vi "(SubVI)DW7802.vi"() -> ()   [LabVIEW 2020]
uses:
  DW7912/Controls/(Ctrl)DW7912_Wave Seq.ctl
  System Command/Controls/(Ctrl)System Command_Trig GPIO Control.ctl
  Register Access/Controls/(Ctrl)Register Access_Cluster.ctl
  <vilib>/Utility/miscctls.llb/LVPointTypeDef.ctl
  Control Data/Controls/(Ctrl)Control Data_Save or Load Control Data_Function.ctl
  Libraries/GUI Log Class/GUI Log Class/Controls/line limit fgv enum.ctl
  Libraries/Haptic IC Class/Haptic IC/Haptic IC.lvclass/Haptic IC.ctl
  I2C/Controls/(Ctrl)I2C_8Bit_Read Array.ctl
  Waveform Editor/Controls/(Ctrl)Waveform Editor_Update Sampling Rate Value.ctl
  b2b9b553-3e13-44b6-91d2-097a3bc441c9.vi
  ce66826c-65e6-4b6c-9d2d-5a99ab5dd81e.vi
  a7fdcbe2-e318-4fc3-ac41-e38a3fe8abb3.vi
  Libraries/Haptic IC Class/Haptic IC/Accessors/Write freq ref.vi
  Libraries/Haptic IC Class/Haptic IC/Accessors/Write voltage range ref.vi
  Libraries/Haptic IC Class/Haptic IC/Accessors/Write mode ref.vi
  Variables/(Var)System Variables.vi
  I2C/Instance VIs/(SubVI)I2C_8Bit-8Bit_Read_Single.vi
  I2C/Instance VIs/(SubVI)I2C_8Bit-8Bit_Read_Sequential.vi
  I2C/Instance VIs/(SubVI)I2C_8Bit-8Bit_Read_Array.vi
  I2C/Instance VIs/(SubVI)I2C_8Bit-8Bit_Write_Single.vi
  I2C/Instance VIs/(SubVI)I2C_8Bit-8Bit_Write_Sequential.vi
  <vilib>/Comparison/Equal/Equal Functor/Equal Functor.lvclass
  Libraries/GUI Log Class/GUI Log Class/GUI Log Class.lvclass
  Libraries/Haptic IC Class/Haptic IC/Haptic IC.lvclass
panel:
  in  "MEM/AT_AB":T1={"OD Cycle"=2, "OD Level"=0, "OD Enable"=TRUE, "Shape"=0, "Enable"=FALSE, "Gain"=0} caption="BRAKE CTRL" {"Gain" items=["Auto", "X1.0", "X0.9", "X0.8", "X0.7", "X0.6", "X0.5", "X0.4"]; "OD Cycle" items=["4 Cycles", "6 Cycles", "8 Cycles", "10 Cycles"]; "OD Level" items=["X1.2", "X1.3", "X1.4", "X1.5"]; "Shape" items=["Square Wave", "Sine Wave"]}
  in  "Stop":bool
  in  "Read All":bool
  in  "Mode Tab":T2(tab)
  in  "Mem Set_Wave Seq Loop":T3 {"Loop 7" items=["X1", "X2", "X3", "X4", "X5", "X6", "X7", "X8", "X9", "X10", "X11", "X12", "X13", "X14", "X15", "Infinite"]; "Loop 6" items=["X1", "X2", "X3", "X4", "X5", "X6", "X7", "X8", "X9", "X10", "X11", "X12", "X13", "X14", "X15", "Infinite"]; "Loop 5" items=["X1", "X2", "X3", "X4", "X5", "X6", "X7", "X8", "X9", "X10", "X11", "X12", "X13", "X14", "X15", "Infinite"]; "Loop 4" items=["X1", "X2", "X3", "X4", "X5", "X6", "X7", "X8", "X9", "X10", "X11", "X12", "X13", "X14", "X15", "Infinite"]; "Loop 3" items=["X1", "X2", "X3", "X4", "X5", "X6", "X7", "X8", "X9", "X10", "X11", "X12", "X13", "X14", "X15", "Infinite"]; "Loop 2" items=["X1", "X2", "X3", "X4", "X5", "X6", "X7", "X8", "X9", "X10", "X11", "X12", "X13", "X14", "X15", "Infinite"]; "Loop 1" items=["X1", "X2", "X3", "X4", "X5", "X6", "X7", "X8", "X9", "X10", "X11", "X12", "X13", "X14", "X15", "Infinite"]; "Loop 0" items=["X1", "X2", "X3", "X4", "X5", "X6", "X7", "X8", "X9", "X10", "X11", "X12", "X13", "X14", "X15", "Infinite"]}
  in  "Mem_Stop":bool
  in  "Mem_Start":bool
  in  "Mem_Wave Seq":T5 caption="WAVE SEQUENCE" {"Wave Seq. 7"."Seq/Delay" items=["Empty", "1", "2", "3", "4", "5", "6", "7", "8", "9", "10", "11", "12", "13", "14", "15", "16", "17", "18", "19", "20", "21", "22", "23", "24", "25", "26", "27", "28", "29", "30", "31", "32", "33", "34", "35", "36", "37", "38", "39", "40", "41", "42", "43", "44", "45", "46", "47", "48", "49", "50", "51", "52", "53", "54", "55", "56", "57", "58", "59", "60", "61", "62", "63", "64", "65", "66", "67", "68", "69", "70", "71", "72", "73", "74", "75", "76", "77", "78", "79", "80", "81", "82", "83", "84", "85", "86", "87", "88", "89", "90", "91", "92", "93", "94", "95", "96", "97", "98", "99", "100", "101", "102", "103", "104", "105", "106", "107", "108", "109", "110", "111", "112", "113", "114", "115", "116", "117", "118", "119", "120", "121", "122", "123", "124", "125", "126", "127"]; "Wave Seq. 7"."Mode" items=["Wave Seq. 7", "Delay"]; "Wave Seq. 6"."Seq/Delay" items=["Empty", "1", "2", "3", "4", "5", "6", "7", "8", "9", "10", "11", "12", "13", "14", "15", "16", "17", "18", "19", "20", "21", "22", "23", "24", "25", "26", "27", "28", "29", "30", "31", "32", "33", "34", "35", "36", "37", "38", "39", "40", "41", "42", "43", "44", "45", "46", "47", "48", "49", "50", "51", "52", "53", "54", "55", "56", "57", "58", "59", "60", "61", "62", "63", "64", "65", "66", "67", "68", "69", "70", "71", "72", "73", "74", "75", "76", "77", "78", "79", "80", "81", "82", "83", "84", "85", "86", "87", "88", "89", "90", "91", "92", "93", "94", "95", "96", "97", "98", "99", "100", "101", "102", "103", "104", "105", "106", "107", "108", "109", "110", "111", "112", "113", "114", "115", "116", "117", "118", "119", "120", "121", "122", "123", "124", "125", "126", "127"]; "Wave Seq. 6"."Mode" items=["Wave Seq. 6", "Delay"]; "Wave Seq. 5"."Seq/Delay" items=["Empty", "1", "2", "3", "4", "5", "6", "7", "8", "9", "10", "11", "12", "13", "14", "15", "16", "17", "18", "19", "20", "21", "22", "23", "24", "25", "26", "27", "28", "29", "30", "31", "32", "33", "34", "35", "36", "37", "38", "39", "40", "41", "42", "43", "44", "45", "46", "47", "48", "49", "50", "51", "52", "53", "54", "55", "56", "57", "58", "59", "60", "61", "62", "63", "64", "65", "66", "67", "68", "69", "70", "71", "72", "73", "74", "75", "76", "77", "78", "79", "80", "81", "82", "83", "84", "85", "86", "87", "88", "89", "90", "91", "92", "93", "94", "95", "96", "97", "98", "99", "100", "101", "102", "103", "104", "105", "106", "107", "108", "109", "110", "111", "112", "113", "114", "115", "116", "117", "118", "119", "120", "121", "122", "123", "124", "125", "126", "127"]; "Wave Seq. 5"."Mode" items=["Wave Seq. 5", "Delay"]; "Wave Seq. 4"."Seq/Delay" items=["Empty", "1", "2", "3", "4", "5", "6", "7", "8", "9", "10", "11", "12", "13", "14", "15", "16", "17", "18", "19", "20", "21", "22", "23", "24", "25", "26", "27", "28", "29", "30", "31", "32", "33", "34", "35", "36", "37", "38", "39", "40", "41", "42", "43", "44", "45", "46", "47", "48", "49", "50", "51", "52", "53", "54", "55", "56", "57", "58", "59", "60", "61", "62", "63", "64", "65", "66", "67", "68", "69", "70", "71", "72", "73", "74", "75", "76", "77", "78", "79", "80", "81", "82", "83", "84", "85", "86", "87", "88", "89", "90", "91", "92", "93", "94", "95", "96", "97", "98", "99", "100", "101", "102", "103", "104", "105", "106", "107", "108", "109", "110", "111", "112", "113", "114", "115", "116", "117", "118", "119", "120", "121", "122", "123", "124", "125", "126", "127"]; "Wave Seq. 4"."Mode" items=["Wave Seq. 4", "Delay"]; "Wave Seq. 3"."Seq/Delay" items=["Empty", "1", "2", "3", "4", "5", "6", "7", "8", "9", "10", "11", "12", "13", "14", "15", "16", "17", "18", "19", "20", "21", "22", "23", "24", "25", "26", "27", "28", "29", "30", "31", "32", "33", "34", "35", "36", "37", "38", "39", "40", "41", "42", "43", "44", "45", "46", "47", "48", "49", "50", "51", "52", "53", "54", "55", "56", "57", "58", "59", "60", "61", "62", "63", "64", "65", "66", "67", "68", "69", "70", "71", "72", "73", "74", "75", "76", "77", "78", "79", "80", "81", "82", "83", "84", "85", "86", "87", "88", "89", "90", "91", "92", "93", "94", "95", "96", "97", "98", "99", "100", "101", "102", "103", "104", "105", "106", "107", "108", "109", "110", "111", "112", "113", "114", "115", "116", "117", "118", "119", "120", "121", "122", "123", "124", "125", "126", "127"]; "Wave Seq. 3"."Mode" items=["Wave Seq. 3", "Delay"]; "Wave Seq. 2"."Seq/Delay" items=["Empty", "1", "2", "3", "4", "5", "6", "7", "8", "9", "10", "11", "12", "13", "14", "15", "16", "17", "18", "19", "20", "21", "22", "23", "24", "25", "26", "27", "28", "29", "30", "31", "32", "33", "34", "35", "36", "37", "38", "39", "40", "41", "42", "43", "44", "45", "46", "47", "48", "49", "50", "51", "52", "53", "54", "55", "56", "57", "58", "59", "60", "61", "62", "63", "64", "65", "66", "67", "68", "69", "70", "71", "72", "73", "74", "75", "76", "77", "78", "79", "80", "81", "82", "83", "84", "85", "86", "87", "88", "89", "90", "91", "92", "93", "94", "95", "96", "97", "98", "99", "100", "101", "102", "103", "104", "105", "106", "107", "108", "109", "110", "111", "112", "113", "114", "115", "116", "117", "118", "119", "120", "121", "122", "123", "124", "125", "126", "127"]; "Wave Seq. 2"."Mode" items=["Wave Seq. 2", "Delay"]; "Wave Seq. 1"."Seq/Delay" items=["Empty", "1", "2", "3", "4", "5", "6", "7", "8", "9", "10", "11", "12", "13", "14", "15", "16", "17", "18", "19", "20", "21", "22", "23", "24", "25", "26", "27", "28", "29", "30", "31", "32", "33", "34", "35", "36", "37", "38", "39", "40", "41", "42", "43", "44", "45", "46", "47", "48", "49", "50", "51", "52", "53", "54", "55", "56", "57", "58", "59", "60", "61", "62", "63", "64", "65", "66", "67", "68", "69", "70", "71", "72", "73", "74", "75", "76", "77", "78", "79", "80", "81", "82", "83", "84", "85", "86", "87", "88", "89", "90", "91", "92", "93", "94", "95", "96", "97", "98", "99", "100", "101", "102", "103", "104", "105", "106", "107", "108", "109", "110", "111", "112", "113", "114", "115", "116", "117", "118", "119", "120", "121", "122", "123", "124", "125", "126", "127"]; "Wave Seq. 1"."Mode" items=["Wave Seq. 1", "Delay"]; "Wave Seq. 0"."Seq/Delay" items=["Empty", "1", "2", "3", "4", "5", "6", "7", "8", "9", "10", "11", "12", "13", "14", "15", "16", "17", "18", "19", "20", "21", "22", "23", "24", "25", "26", "27", "28", "29", "30", "31", "32", "33", "34", "35", "36", "37", "38", "39", "40", "41", "42", "43", "44", "45", "46", "47", "48", "49", "50", "51", "52", "53", "54", "55", "56", "57", "58", "59", "60", "61", "62", "63", "64", "65", "66", "67", "68", "69", "70", "71", "72", "73", "74", "75", "76", "77", "78", "79", "80", "81", "82", "83", "84", "85", "86", "87", "88", "89", "90", "91", "92", "93", "94", "95", "96", "97", "98", "99", "100", "101", "102", "103", "104", "105", "106", "107", "108", "109", "110", "111", "112", "113", "114", "115", "116", "117", "118", "119", "120", "121", "122", "123", "124", "125", "126", "127"]; "Wave Seq. 0"."Mode" items=["Wave Seq. 0", "Delay"]}
  in  "Mem_Main Seq Loop":u8(ring) caption="Sequence Loop" items=["X1", "X2", "X3", "X4", "X5", "X6", "X7", "X8", "X9", "X10", "X11", "X12", "X13", "X14", "X15", "Infinite"]
  in  "Mem_Read":bool caption="Memory Mode"
  in  "Com_Bst_Mem Gain":u8(ring) caption="MEM Gain" items=["100%", "87.5%", "75%", "62.5%", "50%", "37.5%", "25%", "12.5%"]
  in  "Com_Bst_Mute":bool
  in  "AT_Track_OD Cycle":u8(ring)=2 caption="Over Drive Cycle" items=["4 Cycles", "6 Cycles", "8 Cycles", "10 Cycles"]
  in  "AT_Track_OD Level":u8(ring) caption="Over Drive Level" items=["X1.2", "X1.3", "X1.4", "X1.5"]
  in  "AT_Track_OD Enable":bool=TRUE
  in  "AT_Track_Shape":u8(ring) caption="Track Shape" items=["Square Wave", "Sine Wave"]
  in  "AT_Track_Idle":u8(ring)=3 caption="Track Idle" items=["10.66ms", "21.32ms", "31.98ms", "42.64ms", "53.30ms", "63.96ms", "74.62ms", "85.28ms", "95.94ms", "106.60ms", "117.26ms", "127.92ms", "138.58ms", "149.24ms", "159.90ms", "170.56ms", "181.22ms", "191.88ms", "202.54ms", "213.20ms", "223.86ms", "234.52ms", "245.18ms", "255.84ms", "266.50ms", "277.16ms", "287.82ms", "298.48ms", "309.14ms", "319.80ms", "330.46ms", "341.12ms", "351.78ms", "362.44ms", "373.10ms", "383.76ms", "394.42ms", "405.08ms", "415.74ms", "426.40ms", "437.06ms", "447.72ms", "458.38ms", "469.04ms", "479.70ms", "490.36ms", "501.02ms", "511.68ms", "522.34ms", "533.00ms", "543.66ms", "554.32ms", "564.98ms", "575.64ms", "586.30ms", "596.96ms", "607.62ms", "618.28ms", "628.94ms", "639.60ms", "650.26ms", "660.92ms", "671.58ms", "682.24ms", "692.90ms", "703.56ms", "714.22ms", "724.88ms", "735.54ms", "746.20ms", "756.86ms", "767.52ms", "778.18ms", "788.84ms", "799.50ms", "810.16ms", "820.82ms", "831.48ms", "842.14ms", "852.80ms", "863.46ms", "874.12ms", "884.78ms", "895.44ms", "906.10ms", "916.76ms", "927.42ms", "938.08ms", "948.74ms", "959.40ms", "970.06ms", "980.72ms", "991.38ms", "1002.04ms", "1012.70ms", "1023.36ms", "1034.02ms", "1044.68ms", "1055.34ms", "1066.00ms", "1076.66ms", "1087.32ms", "1097.98ms", "1108.64ms", "1119.30ms", "1129.96ms", "1140.62ms", "1151.28ms", "1161.94ms", "1172.60ms", "1183.26ms", "1193.92ms", "1204.58ms", "1215.24ms", "1225.90ms", "1236.56ms", "1247.22ms", "1257.88ms", "1268.54ms", "1279.20ms", "1289.86ms", "1300.52ms", "1311.18ms", "1321.84ms", "1332.50ms", "1343.16ms", "1353.82ms", "1364.48ms", "1375.14ms", "1385.80ms", "1396.46ms", "1407.12ms", "1417.78ms", "1428.44ms", "1439.10ms", "1449.76ms", "1460.42ms", "1471.08ms", "1481.74ms", "1492.40ms", "1503.06ms", "1513.72ms", "1524.38ms", "1535.04ms", "1545.70ms", "1556.36ms", "1567.02ms", "1577.68ms", "1588.34ms", "1599.00ms", "1609.66ms", "1620.32ms", "1630.98ms", "1641.64ms", "1652.30ms", "1662.96ms", "1673.62ms", "1684.28ms", "1694.94ms", "1705.60ms", "1716.26ms", "1726.92ms", "1737.58ms", "1748.24ms", "1758.90ms", "1769.56ms", "1780.22ms", "1790.88ms", "1801.54ms", "1812.20ms", "1822.86ms", "1833.52ms", "1844.18ms", "1854.84ms", "1865.50ms", "1876.16ms", "1886.82ms", "1897.48ms", "1908.14ms", "1918.80ms", "1929.46ms", "1940.12ms", "1950.78ms", "1961.44ms", "1972.10ms", "1982.76ms", "1993.42ms", "2004.08ms", "2014.74ms", "2025.40ms", "2036.06ms", "2046.72ms", "2057.38ms", "2068.04ms", "2078.70ms", "2089.36ms", "2100.02ms", "2110.68ms", "2121.34ms", "2132.00ms", "2142.66ms", "2153.32ms", "2163.98ms", "2174.64ms", "2185.30ms", "2195.96ms", "2206.62ms", "2217.28ms", "2227.94ms", "2238.60ms", "2249.26ms", "2259.92ms", "2270.58ms", "2281.24ms", "2291.90ms", "2302.56ms", "2313.22ms", "2323.88ms", "2334.54ms", "2345.20ms", "2355.86ms", "2366.52ms", "2377.18ms", "2387.84ms", "2398.50ms", "2409.16ms", "2419.82ms", "2430.48ms", "2441.14ms", "2451.80ms", "2462.46ms", "2473.12ms", "2483.78ms", "2494.44ms", "2505.10ms", "2515.76ms", "2526.42ms", "2537.08ms", "2547.74ms", "2558.40ms", "2569.06ms", "2579.72ms", "2590.38ms", "2601.04ms", "2611.70ms", "2622.36ms", "2633.02ms", "2643.68ms", "2654.34ms", "2665.00ms", "2675.66ms", "2686.32ms", "2696.98ms", "2707.64ms", "2718.30ms", "2728.96ms"]
  in  "AT_Track_Play":u8(ring)=128 caption="Track Play" items=["10.66ms", "21.32ms", "31.98ms", "42.64ms", "53.30ms", "63.96ms", "74.62ms", "85.28ms", "95.94ms", "106.60ms", "117.26ms", "127.92ms", "138.58ms", "149.24ms", "159.90ms", "170.56ms", "181.22ms", "191.88ms", "202.54ms", "213.20ms", "223.86ms", "234.52ms", "245.18ms", "255.84ms", "266.50ms", "277.16ms", "287.82ms", "298.48ms", "309.14ms", "319.80ms", "330.46ms", "341.12ms", "351.78ms", "362.44ms", "373.10ms", "383.76ms", "394.42ms", "405.08ms", "415.74ms", "426.40ms", "437.06ms", "447.72ms", "458.38ms", "469.04ms", "479.70ms", "490.36ms", "501.02ms", "511.68ms", "522.34ms", "533.00ms", "543.66ms", "554.32ms", "564.98ms", "575.64ms", "586.30ms", "596.96ms", "607.62ms", "618.28ms", "628.94ms", "639.60ms", "650.26ms", "660.92ms", "671.58ms", "682.24ms", "692.90ms", "703.56ms", "714.22ms", "724.88ms", "735.54ms", "746.20ms", "756.86ms", "767.52ms", "778.18ms", "788.84ms", "799.50ms", "810.16ms", "820.82ms", "831.48ms", "842.14ms", "852.80ms", "863.46ms", "874.12ms", "884.78ms", "895.44ms", "906.10ms", "916.76ms", "927.42ms", "938.08ms", "948.74ms", "959.40ms", "970.06ms", "980.72ms", "991.38ms", "1002.04ms", "1012.70ms", "1023.36ms", "1034.02ms", "1044.68ms", "1055.34ms", "1066.00ms", "1076.66ms", "1087.32ms", "1097.98ms", "1108.64ms", "1119.30ms", "1129.96ms", "1140.62ms", "1151.28ms", "1161.94ms", "1172.60ms", "1183.26ms", "1193.92ms", "1204.58ms", "1215.24ms", "1225.90ms", "1236.56ms", "1247.22ms", "1257.88ms", "1268.54ms", "1279.20ms", "1289.86ms", "1300.52ms", "1311.18ms", "1321.84ms", "1332.50ms", "1343.16ms", "1353.82ms", "1364.48ms", "1375.14ms", "1385.80ms", "1396.46ms", "1407.12ms", "1417.78ms", "1428.44ms", "1439.10ms", "1449.76ms", "1460.42ms", "1471.08ms", "1481.74ms", "1492.40ms", "1503.06ms", "1513.72ms", "1524.38ms", "1535.04ms", "1545.70ms", "1556.36ms", "1567.02ms", "1577.68ms", "1588.34ms", "1599.00ms", "1609.66ms", "1620.32ms", "1630.98ms", "1641.64ms", "1652.30ms", "1662.96ms", "1673.62ms", "1684.28ms", "1694.94ms", "1705.60ms", "1716.26ms", "1726.92ms", "1737.58ms", "1748.24ms", "1758.90ms", "1769.56ms", "1780.22ms", "1790.88ms", "1801.54ms", "1812.20ms", "1822.86ms", "1833.52ms", "1844.18ms", "1854.84ms", "1865.50ms", "1876.16ms", "1886.82ms", "1897.48ms", "1908.14ms", "1918.80ms", "1929.46ms", "1940.12ms", "1950.78ms", "1961.44ms", "1972.10ms", "1982.76ms", "1993.42ms", "2004.08ms", "2014.74ms", "2025.40ms", "2036.06ms", "2046.72ms", "2057.38ms", "2068.04ms", "2078.70ms", "2089.36ms", "2100.02ms", "2110.68ms", "2121.34ms", "2132.00ms", "2142.66ms", "2153.32ms", "2163.98ms", "2174.64ms", "2185.30ms", "2195.96ms", "2206.62ms", "2217.28ms", "2227.94ms", "2238.60ms", "2249.26ms", "2259.92ms", "2270.58ms", "2281.24ms", "2291.90ms", "2302.56ms", "2313.22ms", "2323.88ms", "2334.54ms", "2345.20ms", "2355.86ms", "2366.52ms", "2377.18ms", "2387.84ms", "2398.50ms", "2409.16ms", "2419.82ms", "2430.48ms", "2441.14ms", "2451.80ms", "2462.46ms", "2473.12ms", "2483.78ms", "2494.44ms", "2505.10ms", "2515.76ms", "2526.42ms", "2537.08ms", "2547.74ms", "2558.40ms", "2569.06ms", "2579.72ms", "2590.38ms", "2601.04ms", "2611.70ms", "2622.36ms", "2633.02ms", "2643.68ms", "2654.34ms", "2665.00ms", "2675.66ms", "2686.32ms", "2696.98ms", "2707.64ms", "2718.30ms", "Infinite"]
  in  "AT_Track_Loop":u8(ring) caption="Track Loop" items=["X1", "X2", "X3", "X4", "X5", "X6", "X7", "X8", "X9", "X10", "X11", "X12", "X13", "X14", "X15", "Infinite"]
  in  "AT_Track_Pattern":bool=TRUE
  in  "AT_Read":bool caption="Auto Track Mode"
  in  "AT_Start":bool
  in  "AT_Stop":bool
  in  "Trig_Wave_F_Enable":bool=TRUE
  in  "Trig_Wave_R_Enable":bool=TRUE
  in  "Trig_Wave_F":u8(ring) caption="TRIG F Wave" items=["Empty", "1", "2", "3", "4", "5", "6", "7", "8", "9", "10", "11", "12", "13", "14", "15", "16", "17", "18", "19", "20", "21", "22", "23", "24", "25", "26", "27", "28", "29", "30", "31", "32", "33", "34", "35", "36", "37", "38", "39", "40", "41", "42", "43", "44", "45", "46", "47", "48", "49", "50", "51", "52", "53", "54", "55", "56", "57", "58", "59", "60", "61", "62", "63", "64", "65", "66", "67", "68", "69", "70", "71", "72", "73", "74", "75", "76", "77", "78", "79", "80", "81", "82", "83", "84", "85", "86", "87", "88", "89", "90", "91", "92", "93", "94", "95", "96", "97", "98", "99", "100", "101", "102", "103", "104", "105", "106", "107", "108", "109", "110", "111", "112", "113", "114", "115", "116", "117", "118", "119", "120", "121", "122", "123", "124", "125", "126", "127"]
  in  "Trig_Wave_R":u8(ring) caption="TRIG R Wave" items=["Empty", "1", "2", "3", "4", "5", "6", "7", "8", "9", "10", "11", "12", "13", "14", "15", "16", "17", "18", "19", "20", "21", "22", "23", "24", "25", "26", "27", "28", "29", "30", "31", "32", "33", "34", "35", "36", "37", "38", "39", "40", "41", "42", "43", "44", "45", "46", "47", "48", "49", "50", "51", "52", "53", "54", "55", "56", "57", "58", "59", "60", "61", "62", "63", "64", "65", "66", "67", "68", "69", "70", "71", "72", "73", "74", "75", "76", "77", "78", "79", "80", "81", "82", "83", "84", "85", "86", "87", "88", "89", "90", "91", "92", "93", "94", "95", "96", "97", "98", "99", "100", "101", "102", "103", "104", "105", "106", "107", "108", "109", "110", "111", "112", "113", "114", "115", "116", "117", "118", "119", "120", "121", "122", "123", "124", "125", "126", "127"]
  out "Trig_Gen_Pict":picture
  in  "Trig_Ctrl_Interval":u8(ring)=4 caption="TRIG Interval" items=["2.5ms", "5ms", "10ms", "20ms", "40ms", "60ms", "80ms", "100ms"]
  in  "Trig_Ctrl_Tirg Mode":bool=TRUE
  in  "Trig_Ctrl_Restart Enable":bool
  in  "Trig_Ctrl_Trig Level":bool
  in  "Trig_Ctrl_Trig Priority":bool
  in  "Trig_Gen_Set":bool
  in  "Trig_Gen_Setting":T6={"1st Trig"={"Trigger"=TRUE, "Low"=0, "High"=100}, "2nd Trig"={"Trigger"=FALSE, "Low"=0, "High"=100}, "3rd Trig"={"Trigger"=FALSE, "Low"=0, "High"=100}, "4th Trig"={"Trigger"=FALSE, "Low"=0, "High"=1}} {"4th Trig"."High" min=1 max=8000; "4th Trig"."Low" max=7999; "3rd Trig"."High" min=1 max=8000; "3rd Trig"."Low" max=7999; "2nd Trig"."High" min=1 max=8000; "2nd Trig"."Low" max=7999; "1st Trig"."High" min=1 max=8000; "1st Trig"."Low" max=7999}
  in  "Trig_Read":bool caption="Trig Mode"
  in  "Common Tab":T7(tab)
  in  "Com_ACT_CAL F0":bool
  in  "Com_ACT_F0 In":u16(ring)=180 caption="ACT F0 In" items=["0Hz", "1Hz", "2Hz", "3Hz", "4Hz", "5Hz", "6Hz", "7Hz", "8Hz", "9Hz", "10Hz", "11Hz", "12Hz", "13Hz", "14Hz", "15Hz", "16Hz", "17Hz", "18Hz", "19Hz", "20Hz", "21Hz", "22Hz", "23Hz", "24Hz", "25Hz", "26Hz", "27Hz", "28Hz", "29Hz", "30Hz", "31Hz", "32Hz", "33Hz", "34Hz", "35Hz", "36Hz", "37Hz", "38Hz", "39Hz", "40Hz", "41Hz", "42Hz", "43Hz", "44Hz", "45Hz", "46Hz", "47Hz", "48Hz", "49Hz", "50Hz", "51Hz", "52Hz", "53Hz", "54Hz", "55Hz", "56Hz", "57Hz", "58Hz", "59Hz", "60Hz", "61Hz", "62Hz", "63Hz", "64Hz", "65Hz", "66Hz", "67Hz", "68Hz", "69Hz", "70Hz", "71Hz", "72Hz", "73Hz", "74Hz", "75Hz", "76Hz", "77Hz", "78Hz", "79Hz", "80Hz", "81Hz", "82Hz", "83Hz", "84Hz", "85Hz", "86Hz", "87Hz", "88Hz", "89Hz", "90Hz", "91Hz", "92Hz", "93Hz", "94Hz", "95Hz", "96Hz", "97Hz", "98Hz", "99Hz", "100Hz", "101Hz", "102Hz", "103Hz", "104Hz", "105Hz", "106Hz", "107Hz", "108Hz", "109Hz", "110Hz", "111Hz", "112Hz", "113Hz", "114Hz", "115Hz", "116Hz", "117Hz", "118Hz", "119Hz", "120Hz", "121Hz", "122Hz", "123Hz", "124Hz", "125Hz", "126Hz", "127Hz", "128Hz", "129Hz", "130Hz", "131Hz", "132Hz", "133Hz", "134Hz", "135Hz", "136Hz", "137Hz", "138Hz", "139Hz", "140Hz", "141Hz", "142Hz", "143Hz", "144Hz", "145Hz", "146Hz", "147Hz", "148Hz", "149Hz", "150Hz", "151Hz", "152Hz", "153Hz", "154Hz", "155Hz", "156Hz", "157Hz", "158Hz", "159Hz", "160Hz", "161Hz", "162Hz", "163Hz", "164Hz", "165Hz", "166Hz", "167Hz", "168Hz", "169Hz", "170Hz", "171Hz", "172Hz", "173Hz", "174Hz", "175Hz", "176Hz", "177Hz", "178Hz", "179Hz", "180Hz", "181Hz", "182Hz", "183Hz", "184Hz", "185Hz", "186Hz", "187Hz", "188Hz", "189Hz", "190Hz", "191Hz", "192Hz", "193Hz", "194Hz", "195Hz", "196Hz", "197Hz", "198Hz", "199Hz", "200Hz", "201Hz", "202Hz", "203Hz", "204Hz", "205Hz", "206Hz", "207Hz", "208Hz", "209Hz", "210Hz", "211Hz", "212Hz", "213Hz", "214Hz", "215Hz", "216Hz", "217Hz", "218Hz", "219Hz", "220Hz", "221Hz", "222Hz", "223Hz", "224Hz", "225Hz", "226Hz", "227Hz", "228Hz", "229Hz", "230Hz", "231Hz", "232Hz", "233Hz", "234Hz", "235Hz", "236Hz", "237Hz", "238Hz", "239Hz", "240Hz", "241Hz", "242Hz", "243Hz", "244Hz", "245Hz", "246Hz", "247Hz", "248Hz", "249Hz", "250Hz", "251Hz", "252Hz", "253Hz", "254Hz", "255Hz", "256Hz", "257Hz", "258Hz", "259Hz", "260Hz", "261Hz", "262Hz", "263Hz", "264Hz", "265Hz", "266Hz", "267Hz", "268Hz", "269Hz", "270Hz", "271Hz", "272Hz", "273Hz", "274Hz", "275Hz", "276Hz", "277Hz", "278Hz", "279Hz", "280Hz", "281Hz", "282Hz", "283Hz", "284Hz", "285Hz", "286Hz", "287Hz", "288Hz", "289Hz", "290Hz", "291Hz", "292Hz", "293Hz", "294Hz", "295Hz", "296Hz", "297Hz", "298Hz", "299Hz", "300Hz", "301Hz", "302Hz", "303Hz", "304Hz", "305Hz", "306Hz", "307Hz", "308Hz", "309Hz", "310Hz", "311Hz", "312Hz", "313Hz", "314Hz", "315Hz", "316Hz", "317Hz", "318Hz", "319Hz", "320Hz", "321Hz", "322Hz", "323Hz", "324Hz", "325Hz", "326Hz", "327Hz", "328Hz", "329Hz", "330Hz", "331Hz", "332Hz", "333Hz", "334Hz", "335Hz", "336Hz", "337Hz", "338Hz", "339Hz", "340Hz", "341Hz", "342Hz", "343Hz", "344Hz", "345Hz", "346Hz", "347Hz", "348Hz", "349Hz", "350Hz", "351Hz", "352Hz", "353Hz", "354Hz", "355Hz", "356Hz", "357Hz", "358Hz", "359Hz", "360Hz", "361Hz", "362Hz", "363Hz", "364Hz", "365Hz", "366Hz", "367Hz", "368Hz", "369Hz", "370Hz", "371Hz", "372Hz", "373Hz", "374Hz", "375Hz", "376Hz", "377Hz", "378Hz", "379Hz", "380Hz", "381Hz", "382Hz", "383Hz", "384Hz", "385Hz", "386Hz", "387Hz", "388Hz", "389Hz", "390Hz", "391Hz", "392Hz", "393Hz", "394Hz", "395Hz", "396Hz", "397Hz", "398Hz", "399Hz", "400Hz", "401Hz", "402Hz", "403Hz", "404Hz", "405Hz", "406Hz", "407Hz", "408Hz", "409Hz", "410Hz", "411Hz", "412Hz", "413Hz", "414Hz", "415Hz", "416Hz", "417Hz", "418Hz", "419Hz", "420Hz", "421Hz", "422Hz", "423Hz", "424Hz", "425Hz", "426Hz", "427Hz", "428Hz", "429Hz", "430Hz", "431Hz", "432Hz", "433Hz", "434Hz", "435Hz", "436Hz", "437Hz", "438Hz", "439Hz", "440Hz", "441Hz", "442Hz", "443Hz", "444Hz", "445Hz", "446Hz", "447Hz", "448Hz", "449Hz", "450Hz", "451Hz", "452Hz", "453Hz", "454Hz", "455Hz", "456Hz", "457Hz", "458Hz", "459Hz", "460Hz", "461Hz", "462Hz", "463Hz", "464Hz", "465Hz", "466Hz", "467Hz", "468Hz", "469Hz", "470Hz", "471Hz", "472Hz", "473Hz", "474Hz", "475Hz", "476Hz", "477Hz", "478Hz", "479Hz", "480Hz", "481Hz", "482Hz", "483Hz", "484Hz", "485Hz", "486Hz", "487Hz", "488Hz", "489Hz", "490Hz", "491Hz", "492Hz", "493Hz", "494Hz", "495Hz", "496Hz", "497Hz", "498Hz", "499Hz", "500Hz", "501Hz", "502Hz", "503Hz", "504Hz", "505Hz", "506Hz", "507Hz", "508Hz", "509Hz", "510Hz", "511Hz"]
  in  "Com_ACT_Freq Range":u16(ring)=1 caption="Freq Range" items=["±20%", "±15%", "±10%", "±5%"]
  in  "Com_Mode_Trig Enable":bool
  in  "Com_Mode_Int Enable":bool
  in  "Com_Mode_Play Mode":u8(ring)=2 caption="Play Mode" items=["MEM Mode", "RTP Mode", "Auto Track Mode", "DIAG Mode"]
  out "Com_Status_Result":string caption="Result"
  in  "Com_VD Clamp":u8(ring)=85 caption="VD Clamp" items=["0.000V", "0.024V", "0.048V", "0.072V", "0.096V", "0.120V", "0.144V", "0.168V", "0.192V", "0.216V", "0.240V", "0.264V", "0.288V", "0.312V", "0.336V", "0.360V", "0.384V", "0.408V", "0.432V", "0.456V", "0.480V", "0.504V", "0.528V", "0.552V", "0.576V", "0.600V", "0.624V", "0.648V", "0.672V", "0.696V", "0.720V", "0.744V", "0.768V", "0.792V", "0.816V", "0.840V", "0.864V", "0.888V", "0.912V", "0.936V", "0.960V", "0.984V", "1.008V", "1.032V", "1.056V", "1.080V", "1.104V", "1.128V", "1.152V", "1.176V", "1.200V", "1.224V", "1.248V", "1.272V", "1.296V", "1.320V", "1.344V", "1.368V", "1.392V", "1.416V", "1.440V", "1.464V", "1.488V", "1.512V", "1.536V", "1.560V", "1.584V", "1.608V", "1.632V", "1.656V", "1.680V", "1.704V", "1.728V", "1.752V", "1.776V", "1.800V", "1.824V", "1.848V", "1.872V", "1.896V", "1.920V", "1.944V", "1.968V", "1.992V", "2.016V", "2.040V", "2.064V", "2.088V", "2.112V", "2.136V", "2.160V", "2.184V", "2.208V", "2.232V", "2.256V", "2.280V", "2.304V", "2.328V", "2.352V", "2.376V", "2.400V", "2.424V", "2.448V", "2.472V", "2.496V", "2.520V", "2.544V", "2.568V", "2.592V", "2.616V", "2.640V", "2.664V", "2.688V", "2.712V", "2.736V", "2.760V", "2.784V", "2.808V", "2.832V", "2.856V", "2.880V", "2.904V", "2.928V", "2.952V", "2.976V", "3.000V", "3.024V", "3.048V", "3.072V", "3.096V", "3.120V", "3.144V", "3.168V", "3.192V", "3.216V", "3.240V", "3.264V", "3.288V", "3.312V", "3.336V", "3.360V", "3.384V", "3.408V", "3.432V", "3.456V", "3.480V", "3.504V", "3.528V", "3.552V", "3.576V", "3.600V", "3.624V", "3.648V", "3.672V", "3.696V", "3.720V", "3.744V", "3.768V", "3.792V", "3.816V", "3.840V", "3.864V", "3.888V", "3.912V", "3.936V", "3.960V", "3.984V", "4.008V", "4.032V", "4.056V", "4.080V", "4.104V", "4.128V", "4.152V", "4.176V", "4.200V", "4.224V", "4.248V", "4.272V", "4.296V", "4.320V", "4.344V", "4.368V", "4.392V", "4.416V", "4.440V", "4.464V", "4.488V", "4.512V", "4.536V", "4.560V", "4.584V", "4.608V", "4.632V", "4.656V", "4.680V", "4.704V", "4.728V", "4.752V", "4.776V", "4.800V", "4.824V", "4.848V", "4.872V", "4.896V", "4.920V", "4.944V", "4.968V", "4.992V", "5.016V", "5.040V", "5.064V", "5.088V", "5.112V", "5.136V", "5.160V", "5.184V", "5.208V", "5.232V", "5.256V", "5.280V", "5.304V", "5.328V", "5.352V", "5.376V", "5.400V", "5.424V", "5.448V", "5.472V", "5.496V", "5.520V", "5.544V", "5.568V", "5.592V", "5.616V", "5.640V", "5.664V", "5.688V", "5.712V", "5.736V", "5.760V", "5.784V", "5.808V", "5.832V", "5.856V", "5.880V", "5.904V", "5.928V", "5.952V", "5.976V", "6.000V", "6.024V", "6.048V", "6.072V", "6.096V", "6.120V"]
  in  "Com_PWM_Mode":u8(ring) caption="VD Clamp Reg" items=["Header", "VD Clamp"]
  in  "Com_PWM_Freq":u8(ring)=2 caption="PWM Freq." items=["12kHz", "24kHz", "48kHz", "48kHz"]
  in  "Com_Status_Select":T8(ring) caption="Select"
  in  "Com_Read":bool caption="Common"
  in  "Com 2_Reset_SWRST":bool
  in  "Com 2_FIFO_Empty Level":u16=256 caption="Empty Level" max=6144
  in  "Com 2_FIFO_Full Level":u16=1792 caption="Full Level" max=6144
  in  "Com 2_FIFO_Size":u16=2048 caption="FIFO Size" max=6144
  in  "Com 2_ZXD_Sense Time":u8(ring)=2 caption="Sense Time" items=["50us", "100us", "150us", "200us"]
  in  "Com 2_ZXD_BEMF Gain":u8(ring)=10 caption="BEMF Gain" items=["1x", "2x", "3x", "4x", "5x", "6x", "8x", "10x", "20x", "30x", "40x", "50x", "60x", "80x", "100x", "120x"]
  in  "Com 2_ZXD_GND Time":u8(ring)=3 caption="GND Time" items=["25us", "50us", "75us", "100us", "125us", "150us", "175us", "200us", "225us", "250us", "275us", "300us", "325us", "350us", "375us", "400us"]
  in  "Com 2_ZXD_Null Time":u8(ring)=3 caption="Null Time" items=["25us", "50us", "75us", "100us", "125us", "150us", "175us", "200us", "225us", "250us", "275us", "300us", "325us", "350us", "375us", "400us"]
  in  "Com 2_INTZ":T9={"OCP"=TRUE, "TSD"=TRUE, "UVLO"=TRUE, "FIFO_EMPTY"=TRUE, "FIFO_FULL"=TRUE, "ACT_OPEN"=TRUE, "ACT_SHORT"=TRUE} caption="INTZ_MASK"
  in  "Com 2_Read":bool caption="Common 2"
  in  "Hidden_Register Access":T11={"Register 1"={"Addr"=64, "Name"="TRACK_CONFIG", "Data Size"=1, "R Data"=0, "R Btn"=FALSE, "W Data"=147, "W Btn"=FALSE}, "Register 2"={"Addr"=65, "Name"="BRAKE_CTRL", "Data Size"=1, "R Data"=0, "R Btn"=FALSE, "W Data"=2, "W Btn"=FALSE}, "Register 3"={"Addr"=66, "Name"="BEMF_VTH/VTL", "Data Size"=1, "R Data"=0, "R Btn"=FALSE, "W Data"=17, "W Btn"=FALSE}, "Register 4"={"Addr"=67, "Name"="BEMF_MAX", "Data Size"=1, "R Data"=0, "R Btn"=FALSE, "W Data"=0, "W Btn"=FALSE}, "Register 5"={"Addr"=68, "Name"="BEMF_MIN", "Data Size"=1, "R Data"=0, "R Btn"=FALSE, "W Data"=0, "W Btn"=FALSE}, "Register 6"={"Addr"=69, "Name"="VCOM", "Data Size"=1, "R Data"=0, "R Btn"=FALSE, "W Data"=0, "W Btn"=FALSE}, "Register 7"={"Addr"=70, "Name"="ACT_CNT", "Data Size"=2, "R Data"=0, "R Btn"=FALSE, "W Data"=0, "W Btn"=FALSE}, "Register 8"={"Addr"=72, "Name"="QTZ_CNT", "Data Size"=2, "R Data"=0, "R Btn"=FALSE, "W Data"=0, "W Btn"=FALSE}, "Register 9"={"Addr"=74, "Name"="ACT_RES_M", "Data Size"=2, "R Data"=0, "R Btn"=FALSE, "W Data"=0, "W Btn"=FALSE}, "Register 10"={"Addr"=76, "Name"="REF_RES", "Data Size"=2, "R Data"=0, "R Btn"=FALSE, "W Data"=0, "W Btn"=FALSE}, "Register 11"={"Addr"=78, "Name"="PROTECTION_ON", "Data Size"=1, "R Data"=0, "R Btn"=FALSE, "W Data"=2, "W Btn"=FALSE}, "Register 12"={"Addr"=79, "Name"="PROTECTION_OFF", "Data Size"=1, "R Data"=0, "R Btn"=FALSE, "W Data"=120, "W Btn"=FALSE}, "Register 13"={"Addr"=0, "Name"="", "Data Size"=1, "R Data"=0, "R Btn"=FALSE, "W Data"=0, "W Btn"=FALSE}, "Register 14"={"Addr"=96, "Name"="TRACK_CONFIG", "Data Size"=1, "R Data"=0, "R Btn"=FALSE, "W Data"=3, "W Btn"=FALSE}, "Register 15"={"Addr"=97, "Name"="BRAKE_CTRL", "Data Size"=1, "R Data"=0, "R Btn"=FALSE, "W Data"=2, "W Btn"=FALSE}, "Register 16"={"Addr"=98, "Name"="HB_CTRL", "Data Size"=1, "R Data"=0, "R Btn"=FALSE, "W Data"=0, "W Btn"=FALSE}, "Register 17"={"Addr"=99, "Name"="BEMF_MAX", "Data Size"=1, "R Data"=0, "R Btn"=FALSE, "W Data"=0, "W Btn"=FALSE}, "Register 18"={"Addr"=100, "Name"="BEMF_MIN", "Data Size"=1, "R Data"=0, "R Btn"=FALSE, "W Data"=0, "W Btn"=FALSE}, "Register 19"={"Addr"=101, "Name"="VCOM", "Data Size"=1, "R Data"=0, "R Btn"=FALSE, "W Data"=0, "W Btn"=FALSE}, "Register 20"={"Addr"=102, "Name"="ACT_CNT", "Data Size"=2, "R Data"=0, "R Btn"=FALSE, "W Data"=0, "W Btn"=FALSE}, "Register 21"={"Addr"=104, "Name"="QTZ_CNT", "Data Size"=2, "R Data"=0, "R Btn"=FALSE, "W Data"=0, "W Btn"=FALSE}, "Register 22"={"Addr"=0, "Name"="", "Data Size"=1, "R Data"=0, "R Btn"=FALSE, "W Data"=0, "W Btn"=FALSE}, "Register 23"={"Addr"=0, "Name"="", "Data Size"=1, "R Data"=0, "R Btn"=FALSE, "W Data"=0, "W Btn"=FALSE}, "Register 24"={"Addr"=0, "Name"="", "Data Size"=1, "R Data"=0, "R Btn"=FALSE, "W Data"=0, "W Btn"=FALSE}} {"Register 24"."W Data" max=255 format="%02x"; "Register 24"."R Data" format="%02x"; "Register 24"."Data Size" items=["8bit"=1, "16bit"=2]; "Register 24"."Addr" format="%02x"; "Register 23"."W Data" max=255 format="%02x"; "Register 23"."R Data" format="%02x"; "Register 23"."Data Size" items=["8bit"=1, "16bit"=2]; "Register 23"."Addr" format="%02x"; "Register 22"."W Data" max=255 format="%02x"; "Register 22"."R Data" format="%02x"; "Register 22"."Data Size" items=["8bit"=1, "16bit"=2]; "Register 22"."Addr" format="%02x"; "Register 21"."W Data" format="%04x"; "Register 21"."R Data" format="%04x"; "Register 21"."Data Size" items=["8bit"=1, "16bit"=2]; "Register 21"."Addr" format="%02x"; "Register 20"."W Data" format="%04x"; "Register 20"."R Data" format="%04x"; "Register 20"."Data Size" items=["8bit"=1, "16bit"=2]; "Register 20"."Addr" format="%02x"; "Register 19"."W Data" max=255 format="%02x"; "Register 19"."R Data" format="%02x"; "Register 19"."Data Size" items=["8bit"=1, "16bit"=2]; "Register 19"."Addr" format="%02x"; "Register 18"."W Data" max=255 format="%02x"; "Register 18"."R Data" format="%02x"; "Register 18"."Data Size" items=["8bit"=1, "16bit"=2]; "Register 18"."Addr" format="%02x"; "Register 17"."W Data" max=255 format="%02x"; "Register 17"."R Data" format="%02x"; "Register 17"."Data Size" items=["8bit"=1, "16bit"=2]; "Register 17"."Addr" format="%02x"; "Register 16"."W Data" max=255 format="%02x"; "Register 16"."R Data" format="%02x"; "Register 16"."Data Size" items=["8bit"=1, "16bit"=2]; "Register 16"."Addr" format="%02x"; "Register 15"."W Data" max=255 format="%02x"; "Register 15"."R Data" format="%02x"; "Register 15"."Data Size" items=["8bit"=1, "16bit"=2]; "Register 15"."Addr" format="%02x"; "Register 14"."W Data" max=255 format="%02x"; "Register 14"."R Data" format="%02x"; "Register 14"."Data Size" items=["8bit"=1, "16bit"=2]; "Register 14"."Addr" format="%02x"; "Register 13"."W Data" max=255 format="%02x"; "Register 13"."R Data" format="%02x"; "Register 13"."Data Size" items=["8bit"=1, "16bit"=2]; "Register 13"."Addr" format="%02x"; "Register 12"."W Data" max=255 format="%02x"; "Register 12"."R Data" format="%02x"; "Register 12"."Data Size" items=["8bit"=1, "16bit"=2]; "Register 12"."Addr" format="%02x"; "Register 11"."W Data" max=255 format="%02x"; "Register 11"."R Data" format="%02x"; "Register 11"."Data Size" items=["8bit"=1, "16bit"=2]; "Register 11"."Addr" format="%02x"; "Register 10"."W Data" format="%04x"; "Register 10"."R Data" format="%04x"; "Register 10"."Data Size" items=["8bit"=1, "16bit"=2]; "Register 10"."Addr" format="%02x"; "Register 9"."W Data" format="%04x"; "Register 9"."R Data" format="%04x"; "Register 9"."Data Size" items=["8bit"=1, "16bit"=2]; "Register 9"."Addr" format="%02x"; "Register 8"."W Data" format="%04x"; "Register 8"."R Data" format="%04x"; "Register 8"."Data Size" items=["8bit"=1, "16bit"=2]; "Register 8"."Addr" format="%02x"; "Register 7"."W Data" format="%04x"; "Register 7"."R Data" format="%04x"; "Register 7"."Data Size" items=["8bit"=1, "16bit"=2]; "Register 7"."Addr" format="%02x"; "Register 6"."W Data" max=255 format="%02x"; "Register 6"."R Data" format="%02x"; "Register 6"."Data Size" items=["8bit"=1, "16bit"=2]; "Register 6"."Addr" format="%02x"; "Register 5"."W Data" max=255 format="%02x"; "Register 5"."R Data" format="%02x"; "Register 5"."Data Size" items=["8bit"=1, "16bit"=2]; "Register 5"."Addr" format="%02x"; "Register 4"."W Data" max=255 format="%02x"; "Register 4"."R Data" format="%02x"; "Register 4"."Data Size" items=["8bit"=1, "16bit"=2]; "Register 4"."Addr" format="%02x"; "Register 3"."W Data" max=255 format="%02x"; "Register 3"."R Data" format="%02x"; "Register 3"."Data Size" items=["8bit"=1, "16bit"=2]; "Register 3"."Addr" format="%02x"; "Register 2"."W Data" max=255 format="%02x"; "Register 2"."R Data" format="%02x"; "Register 2"."Data Size" items=["8bit"=1, "16bit"=2]; "Register 2"."Addr" format="%02x"; "Register 1"."W Data" max=255 format="%02x"; "Register 1"."R Data" format="%02x"; "Register 1"."Data Size" items=["8bit"=1, "16bit"=2]; "Register 1"."Addr" format="%02x"}
  in  "Fuse_Register Access":T11={"Register 1"={"Addr"=144, "Name"="Q0 (CHIP_ID)", "Data Size"=1, "R Data"=0, "R Btn"=FALSE, "W Data"=0, "W Btn"=FALSE}, "Register 2"={"Addr"=145, "Name"="Q1 (F_ACT_F0_IN)", "Data Size"=2, "R Data"=0, "R Btn"=FALSE, "W Data"=0, "W Btn"=FALSE}, "Register 3"={"Addr"=147, "Name"="Q3 (F_REF_RES", "Data Size"=2, "R Data"=0, "R Btn"=FALSE, "W Data"=0, "W Btn"=FALSE}, "Register 4"={"Addr"=149, "Name"="Q5 (CAL)", "Data Size"=2, "R Data"=0, "R Btn"=FALSE, "W Data"=0, "W Btn"=FALSE}, "Register 5"={"Addr"=151, "Name"="Q7 (WEEK)", "Data Size"=1, "R Data"=0, "R Btn"=FALSE, "W Data"=0, "W Btn"=FALSE}, "Register 6"={"Addr"=152, "Name"="Q8 (BEMF)", "Data Size"=1, "R Data"=0, "R Btn"=FALSE, "W Data"=0, "W Btn"=FALSE}, "Register 7"={"Addr"=153, "Name"="Q9 (REG / BEMF)", "Data Size"=1, "R Data"=0, "R Btn"=FALSE, "W Data"=0, "W Btn"=FALSE}, "Register 8"={"Addr"=154, "Name"="Q10 (HB)", "Data Size"=1, "R Data"=0, "R Btn"=FALSE, "W Data"=0, "W Btn"=FALSE}, "Register 9"={"Addr"=155, "Name"="Q11 (ADC)", "Data Size"=1, "R Data"=0, "R Btn"=FALSE, "W Data"=0, "W Btn"=FALSE}, "Register 10"={"Addr"=156, "Name"="Q12 (ADC)", "Data Size"=1, "R Data"=0, "R Btn"=FALSE, "W Data"=0, "W Btn"=FALSE}, "Register 11"={"Addr"=157, "Name"="Q13 (ADC)", "Data Size"=1, "R Data"=0, "R Btn"=FALSE, "W Data"=0, "W Btn"=FALSE}, "Register 12"={"Addr"=158, "Name"="Q14 (ANA)", "Data Size"=1, "R Data"=0, "R Btn"=FALSE, "W Data"=0, "W Btn"=FALSE}, "Register 13"={"Addr"=159, "Name"="Q15 (ANA)", "Data Size"=1, "R Data"=0, "R Btn"=FALSE, "W Data"=0, "W Btn"=FALSE}, "Register 14"={"Addr"=160, "Name"="TM0", "Data Size"=1, "R Data"=0, "R Btn"=FALSE, "W Data"=0, "W Btn"=FALSE}, "Register 15"={"Addr"=161, "Name"="TM1", "Data Size"=1, "R Data"=0, "R Btn"=FALSE, "W Data"=0, "W Btn"=FALSE}, "Register 16"={"Addr"=162, "Name"="TM2", "Data Size"=1, "R Data"=0, "R Btn"=FALSE, "W Data"=0, "W Btn"=FALSE}, "Register 17"={"Addr"=163, "Name"="TM3", "Data Size"=1, "R Data"=0, "R Btn"=FALSE, "W Data"=0, "W Btn"=FALSE}, "Register 18"={"Addr"=164, "Name"="TM4", "Data Size"=2, "R Data"=0, "R Btn"=FALSE, "W Data"=0, "W Btn"=FALSE}, "Register 19"={"Addr"=166, "Name"="TM6", "Data Size"=1, "R Data"=0, "R Btn"=FALSE, "W Data"=0, "W Btn"=FALSE}, "Register 20"={"Addr"=167, "Name"="TM7", "Data Size"=1, "R Data"=0, "R Btn"=FALSE, "W Data"=0, "W Btn"=FALSE}, "Register 21"={"Addr"=168, "Name"="TM8", "Data Size"=1, "R Data"=0, "R Btn"=FALSE, "W Data"=0, "W Btn"=FALSE}, "Register 22"={"Addr"=174, "Name"="PROTECTION_ON", "Data Size"=1, "R Data"=0, "R Btn"=FALSE, "W Data"=120, "W Btn"=FALSE}, "Register 23"={"Addr"=175, "Name"="PROTECTION_OFF", "Data Size"=1, "R Data"=0, "R Btn"=FALSE, "W Data"=2, "W Btn"=FALSE}, "Register 24"={"Addr"=0, "Name"="", "Data Size"=1, "R Data"=0, "R Btn"=FALSE, "W Data"=0, "W Btn"=FALSE}} {"Register 24"."W Data" max=255 format="%02x"; "Register 24"."R Data" format="%02x"; "Register 24"."Data Size" items=["8bit"=1, "16bit"=2]; "Register 24"."Addr" format="%02x"; "Register 23"."W Data" max=255 format="%02x"; "Register 23"."R Data" format="%02x"; "Register 23"."Data Size" items=["8bit"=1, "16bit"=2]; "Register 23"."Addr" format="%02x"; "Register 22"."W Data" max=255 format="%02x"; "Register 22"."R Data" format="%02x"; "Register 22"."Data Size" items=["8bit"=1, "16bit"=2]; "Register 22"."Addr" format="%02x"; "Register 21"."W Data" max=255 format="%02x"; "Register 21"."R Data" format="%02x"; "Register 21"."Data Size" items=["8bit"=1, "16bit"=2]; "Register 21"."Addr" format="%02x"; "Register 20"."W Data" max=255 format="%02x"; "Register 20"."R Data" format="%02x"; "Register 20"."Data Size" items=["8bit"=1, "16bit"=2]; "Register 20"."Addr" format="%02x"; "Register 19"."W Data" max=255 format="%02x"; "Register 19"."R Data" format="%02x"; "Register 19"."Data Size" items=["8bit"=1, "16bit"=2]; "Register 19"."Addr" format="%02x"; "Register 18"."W Data" format="%04x"; "Register 18"."R Data" format="%04x"; "Register 18"."Data Size" items=["8bit"=1, "16bit"=2]; "Register 18"."Addr" format="%02x"; "Register 17"."W Data" max=255 format="%02x"; "Register 17"."R Data" format="%02x"; "Register 17"."Data Size" items=["8bit"=1, "16bit"=2]; "Register 17"."Addr" format="%02x"; "Register 16"."W Data" max=255 format="%02x"; "Register 16"."R Data" format="%02x"; "Register 16"."Data Size" items=["8bit"=1, "16bit"=2]; "Register 16"."Addr" format="%02x"; "Register 15"."W Data" max=255 format="%02x"; "Register 15"."R Data" format="%02x"; "Register 15"."Data Size" items=["8bit"=1, "16bit"=2]; "Register 15"."Addr" format="%02x"; "Register 14"."W Data" max=255 format="%02x"; "Register 14"."R Data" format="%02x"; "Register 14"."Data Size" items=["8bit"=1, "16bit"=2]; "Register 14"."Addr" format="%02x"; "Register 13"."W Data" max=255 format="%02x"; "Register 13"."R Data" format="%02x"; "Register 13"."Data Size" items=["8bit"=1, "16bit"=2]; "Register 13"."Addr" format="%02x"; "Register 12"."W Data" max=255 format="%02x"; "Register 12"."R Data" format="%02x"; "Register 12"."Data Size" items=["8bit"=1, "16bit"=2]; "Register 12"."Addr" format="%02x"; "Register 11"."W Data" max=255 format="%02x"; "Register 11"."R Data" format="%02x"; "Register 11"."Data Size" items=["8bit"=1, "16bit"=2]; "Register 11"."Addr" format="%02x"; "Register 10"."W Data" max=255 format="%02x"; "Register 10"."R Data" format="%02x"; "Register 10"."Data Size" items=["8bit"=1, "16bit"=2]; "Register 10"."Addr" format="%02x"; "Register 9"."W Data" max=255 format="%02x"; "Register 9"."R Data" format="%02x"; "Register 9"."Data Size" items=["8bit"=1, "16bit"=2]; "Register 9"."Addr" format="%02x"; "Register 8"."W Data" max=255 format="%02x"; "Register 8"."R Data" format="%02x"; "Register 8"."Data Size" items=["8bit"=1, "16bit"=2]; "Register 8"."Addr" format="%02x"; "Register 7"."W Data" max=255 format="%02x"; "Register 7"."R Data" format="%02x"; "Register 7"."Data Size" items=["8bit"=1, "16bit"=2]; "Register 7"."Addr" format="%02x"; "Register 6"."W Data" max=255 format="%02x"; "Register 6"."R Data" format="%02x"; "Register 6"."Data Size" items=["8bit"=1, "16bit"=2]; "Register 6"."Addr" format="%02x"; "Register 5"."W Data" max=255 format="%02x"; "Register 5"."R Data" format="%02x"; "Register 5"."Data Size" items=["8bit"=1, "16bit"=2]; "Register 5"."Addr" format="%02x"; "Register 4"."W Data" format="%04x"; "Register 4"."R Data" format="%04x"; "Register 4"."Data Size" items=["8bit"=1, "16bit"=2]; "Register 4"."Addr" format="%02x"; "Register 3"."W Data" format="%04x"; "Register 3"."R Data" format="%04x"; "Register 3"."Data Size" items=["8bit"=1, "16bit"=2]; "Register 3"."Addr" format="%02x"; "Register 2"."W Data" format="%04x"; "Register 2"."R Data" format="%04x"; "Register 2"."Data Size" items=["8bit"=1, "16bit"=2]; "Register 2"."Addr" format="%02x"; "Register 1"."W Data" max=255 format="%02x"; "Register 1"."R Data" format="%02x"; "Register 1"."Data Size" items=["8bit"=1, "16bit"=2]; "Register 1"."Addr" format="%02x"}
  in  "Script_Run Btn":T12
  in  "Script_Path":T13
  # "WAVE SEQ CTRL"
  # "Wave Seq."
  # "Mem No."
  # "Loop"
  # "TRACK CTRL"
  # "TRIG CTRL"
  # "TRIG WAVE CTRL"
  # "TRIGGER GENERATOR"
  # "Trigger"
  # "R (ms)"
  # "F (ms)"
  # "STATUS READ"
  # "MODE"
  # "PWM FREQ / ETC"
  # "VD CLAMP"
  # "ACT CTRL"
  # "ZXD CTRL"
  # "FIFO"
  # "RESET"
  # "Address"
  # "Name"
  # "Size"
  # "Read"
  # "Write"
  # "Address"
  # "Name"
  # "Size"
  # "Read"
  # "Write"
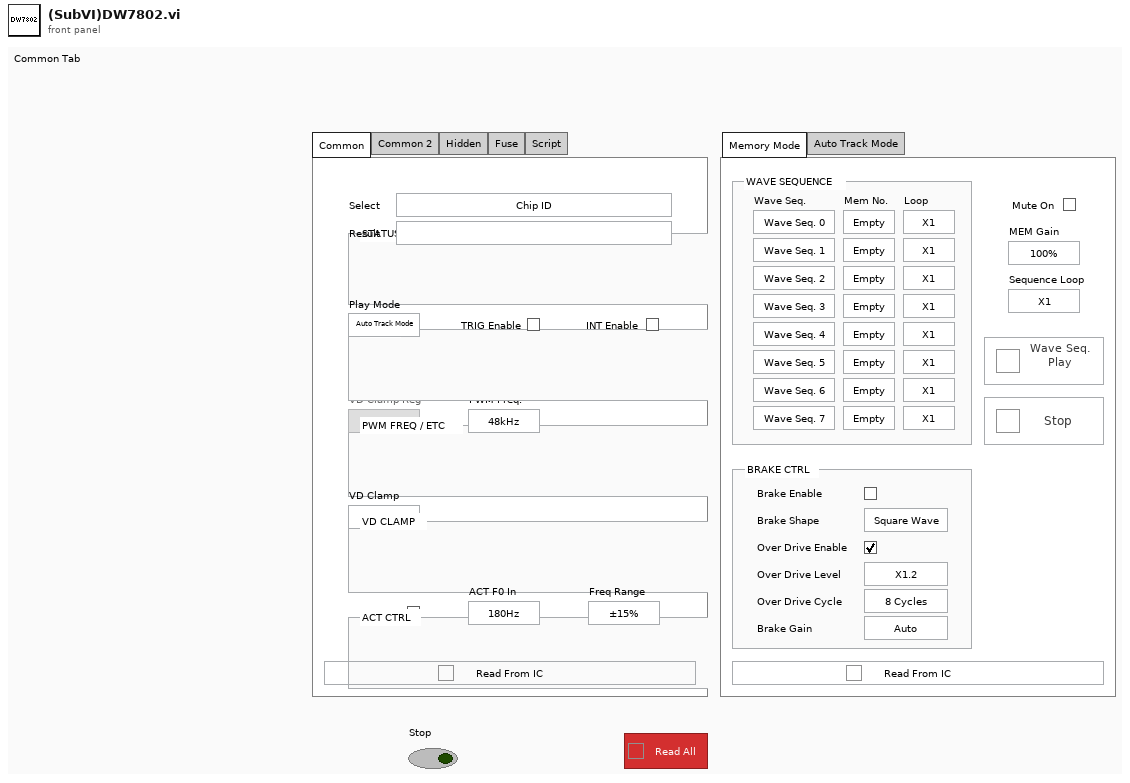
[diagram p1: front panel]
types:
  T1 = cluster{"OD Cycle":u8, "OD Level":u8, "OD Enable":bool, "Shape":u8, "Enable":bool, "Gain":u8}
  T2 = enum32{"Memory Mode", "Auto Track Mode", "Trig Mode"}
  T3 = cluster{"Loop 0":u8, "Loop 1":u8, "Loop 2":u8, "Loop 3":u8, "Loop 4":u8, "Loop 5":u8, "Loop 6":u8, "Loop 7":u8}
  T4 = typedef "(Ctrl)DW7912_Wave Seq.ctl" = cluster{"Mode":u8, "Seq/Delay":u8}
  T5 = cluster{"Wave Seq. 0":T4, "Wave Seq. 1":T4, "Wave Seq. 2":T4, "Wave Seq. 3":T4, "Wave Seq. 4":T4, "Wave Seq. 5":T4, "Wave Seq. 6":T4, "Wave Seq. 7":T4}
  T6 = typedef "(Ctrl)System Command_Trig GPIO Control.ctl" = cluster{"1st Trig":cluster{"Trigger":bool, "Low":u16, "High":u16}, "2nd Trig":cluster{"Trigger":bool, "Low":u16, "High":u16}, "3rd Trig":cluster{"Trigger":bool, "Low":u16, "High":u16}, "4th Trig":cluster{"Trigger":bool, "Low":u16, "High":u16}}
  T7 = enum32{"Common", "Common 2", "Hidden", "Fuse", "Script"}
  T8 = enum16{"Chip ID", "VBAT", "Status", "ACT F0 Value", "FIFO Status", "FIFO Full Level", "FIFO Empty Level", "ACT Resistance", "BEMF Status", ""}
  T9 = cluster{"OCP":bool, "TSD":bool, "UVLO":bool, "FIFO_EMPTY":bool, "FIFO_FULL":bool, "ACT_OPEN":bool, "ACT_SHORT":bool}
  T10 = typedef "(Ctrl)Register Access_Cluster.ctl" = cluster{"Addr":u8, "Name":string, "Data Size":u16, "R Data":u16, "R Btn":bool, "W Data":u16, "W Btn":bool}
  T11 = cluster{"Register 1":T10, "Register 2":T10, "Register 3":T10, "Register 4":T10, "Register 5":T10, "Register 6":T10, "Register 7":T10, "Register 8":T10, "Register 9":T10, "Register 10":T10, "Register 11":T10, "Register 12":T10, "Register 13":T10, "Register 14":T10, "Register 15":T10, "Register 16":T10, "Register 17":T10, "Register 18":T10, "Register 19":T10, "Register 20":T10, "Register 21":T10, "Register 22":T10, "Register 23":T10, "Register 24":T10}
  T12 = cluster{"Run 0":bool, "Run 1":bool, "Run 2":bool, "Run 3":bool, "Run 4":bool, "Run 5":bool, "Run 6":bool, "Run 7":bool, "Run 8":bool, "Run 9":bool, "Run 10":bool, "Run 11":bool, "Run 12":bool, "Run 13":bool, "Run 14":bool, "Run 15":bool, "Run 16":bool, "Run 17":bool, "Run 18":bool, "Run 19":bool, "Run 20":bool, "Run 21":bool, "Run 22":bool, "Run 23":bool}
  T13 = cluster{"Path 1":path, "Path 2":path, "Path 3":path, "Path 4":path, "Path 5":path, "Path 6":path, "Path 7":path, "Path 8":path, "Path 9":path, "Path 10":path, "Path 11":path, "Path 12":path, "Path 13":path, "Path 14":path, "Path 15":path, "Path 16":path, "Path 17":path, "Path 18":path, "Path 19":path, "Path 20":path, "Path 21":path, "Path 22":path, "Path 23":path, "Path 24":path}
  T14 = typedef "GUI Log Class.lvclass/line limit fgv enum.ctl" = enum16{"Read", "Write"}
  T15 = enum8{"Enabled", "Disabled", "Disabled and Grayed Out"}
  T16 = typedef "(Ctrl)Control Data_Save or Load Control Data_Function.ctl" = enum16{"Save", "Load"}
  T17 = typedef "LVPointTypeDef.ctl" = cluster{"Horizontal":i16, "Vertical":i16}
  T18 = enum16{"CHIP ID", "VBAT", "STATUS 0", "STATUS 1", "LRA F0 VALUE", "FIFO STATUS", "RAM CHECKSUM", "FIFO LEVEL"}
  T19 = typedef "(Ctrl)I2C_8Bit_Read Array.ctl" = cluster{"Address":u8, "Delay(ms)":i32}
  T20 = typedef "(Ctrl)Waveform Editor_Update Sampling Rate Value.ctl" = enum16{"Init", "Update"}
  T21 = cluster{"Boolean array[0]":bool, "Boolean array[1]":bool, "Boolean array[2]":bool, "Boolean array[3]":bool, "Boolean array[4]":bool, "Boolean array[5]":bool, "Boolean array[6]":bool}
  T22 = cluster{"[0]":cluster{u8, u8}, "[1]":cluster{u8, u8}, "[2]":cluster{u8, u8}, "[3]":cluster{u8, u8}, "[4]":cluster{u8, u8}, "[5]":cluster{u8, u8}, "[6]":cluster{u8, u8}, "[7]":cluster{u8, u8}}
  T23 = cluster{"[0]":u8, "[1]":u8, "[2]":u8, "[3]":u8, "[4]":u8, "[5]":u8, "[6]":u8, "[7]":u8}
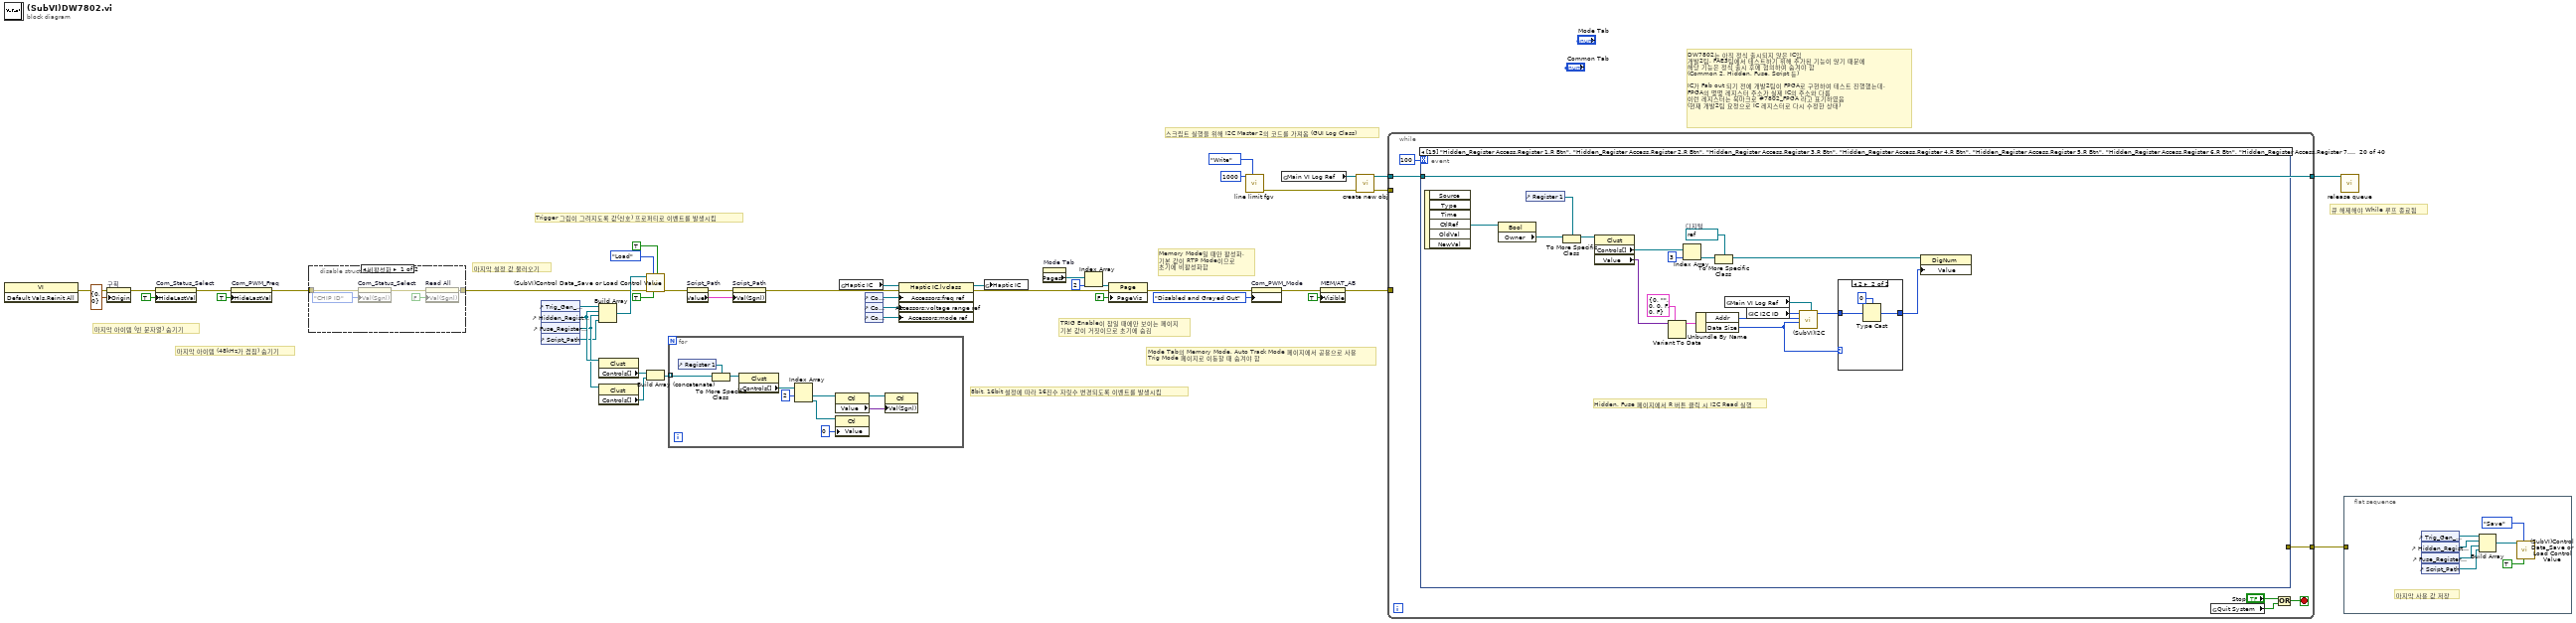
[diagram p0: block diagram]
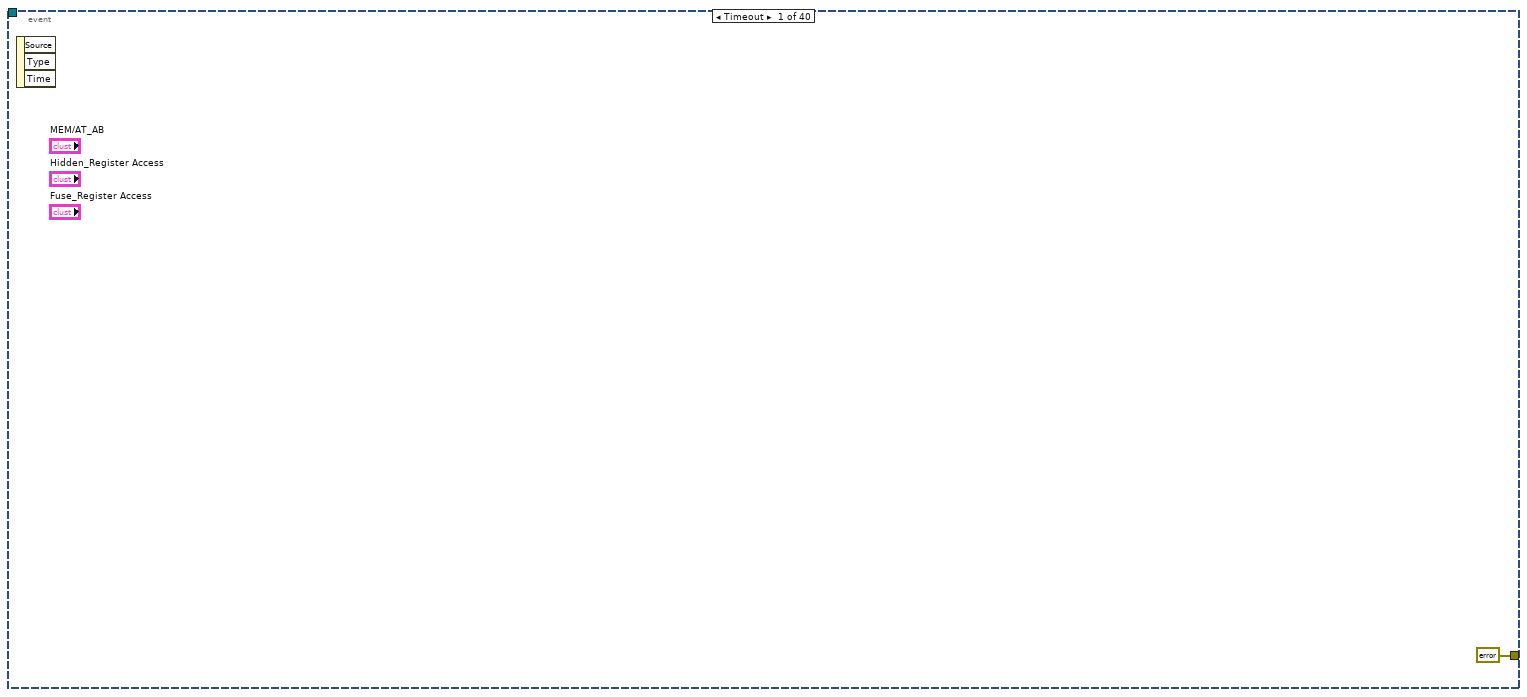
[diagram p3: hidden frame]
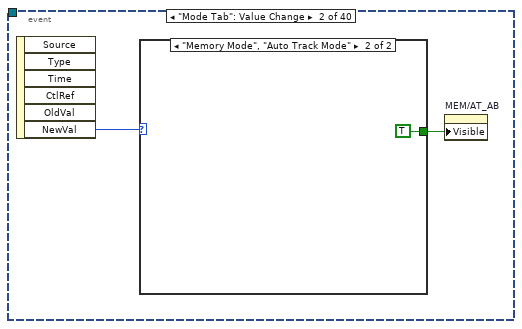
[diagram p4: hidden frame]
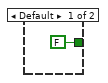
[diagram p5: hidden frame]
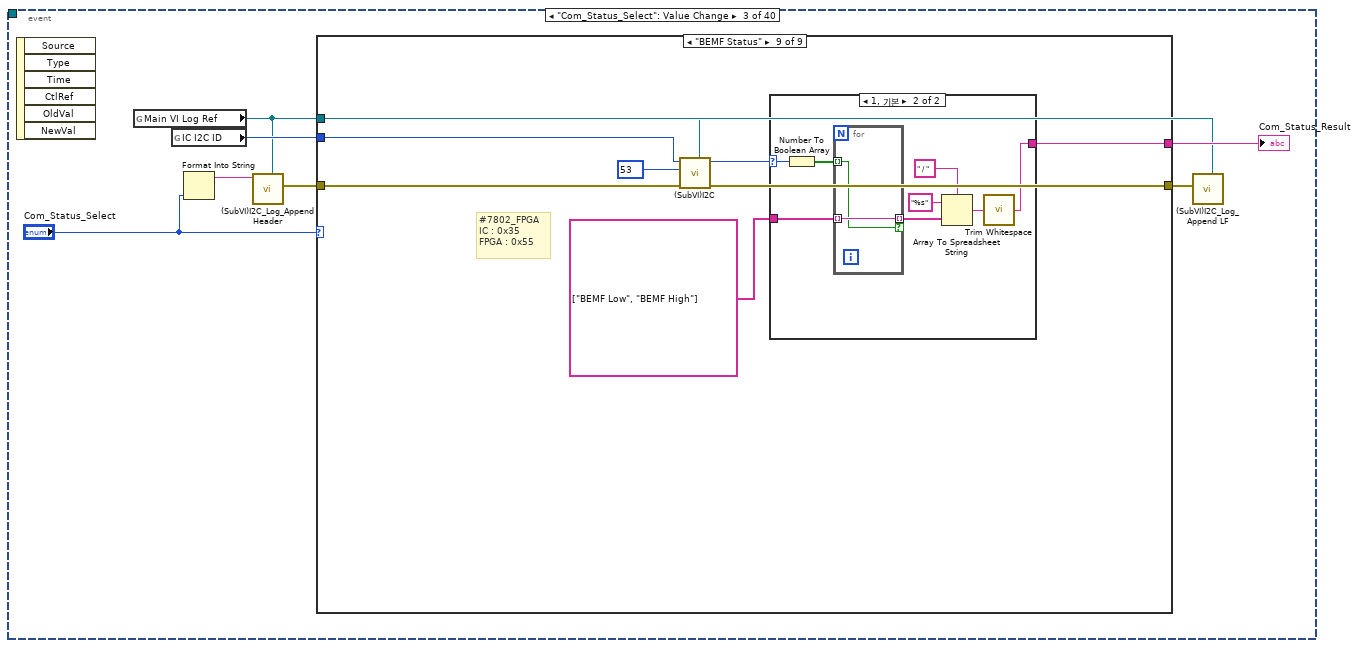
[diagram p6: hidden frame]
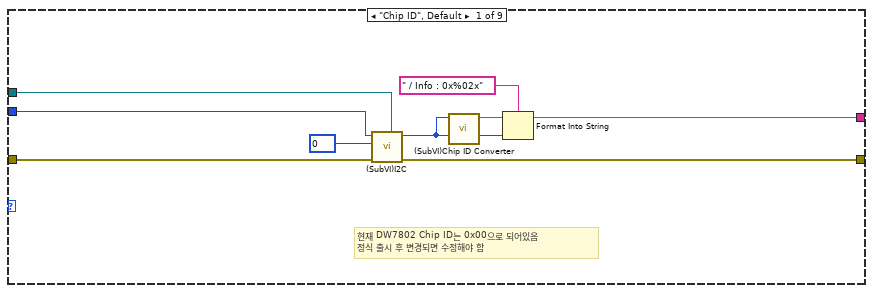
[diagram p7: hidden frame]
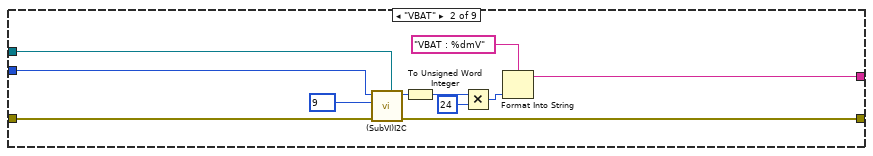
[diagram p8: hidden frame]
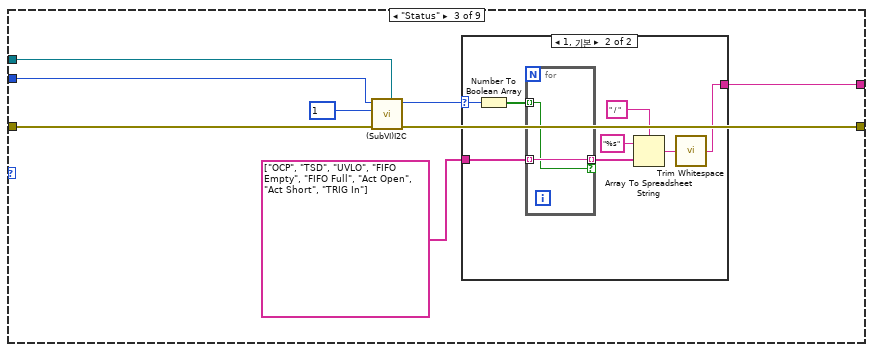
[diagram p9: hidden frame]
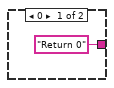
[diagram p10: hidden frame]
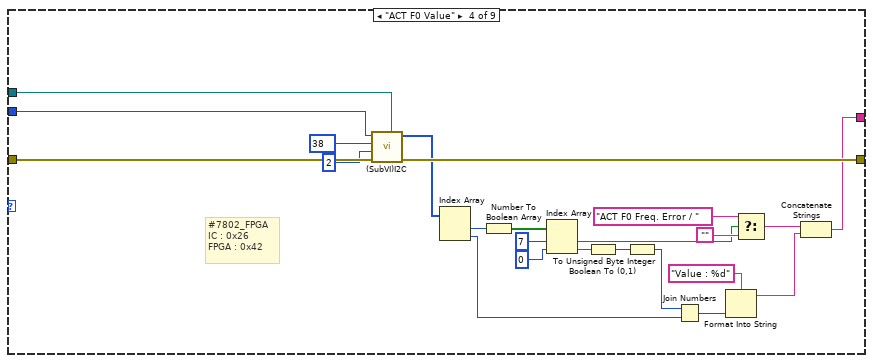
[diagram p11: hidden frame]
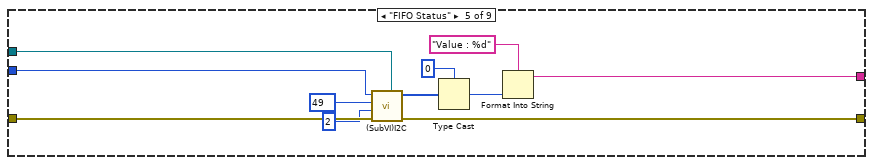
[diagram p12: hidden frame]
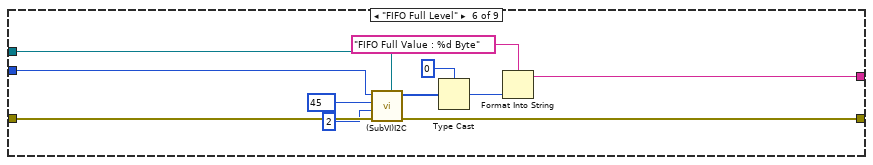
[diagram p13: hidden frame]
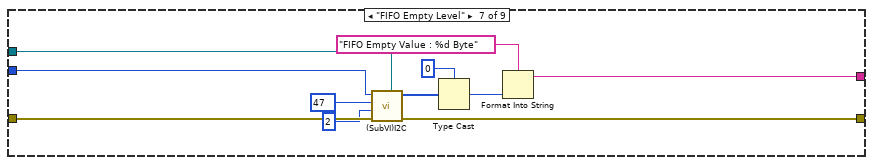
[diagram p14: hidden frame]
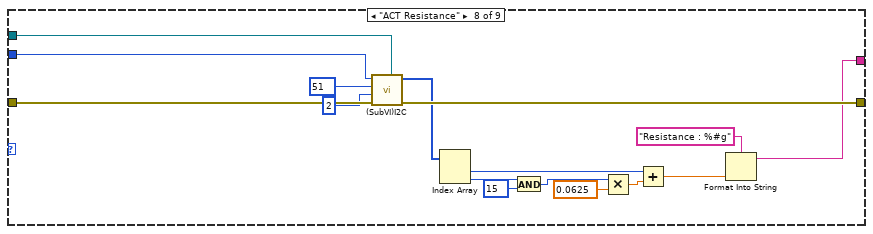
[diagram p15: hidden frame]
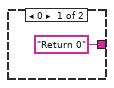
[diagram p16: hidden frame]
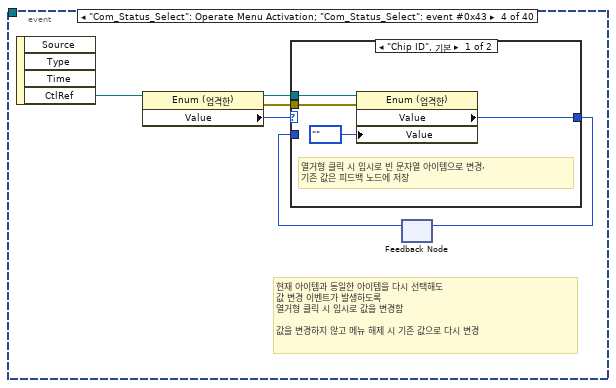
[diagram p17: hidden frame]
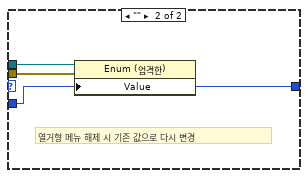
[diagram p18: hidden frame]
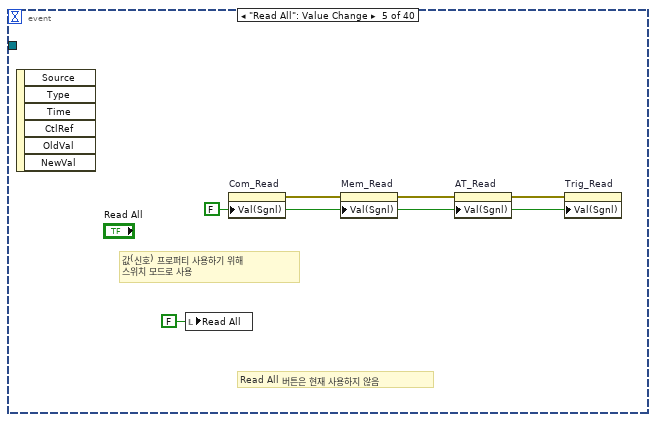
[diagram p19: hidden frame]
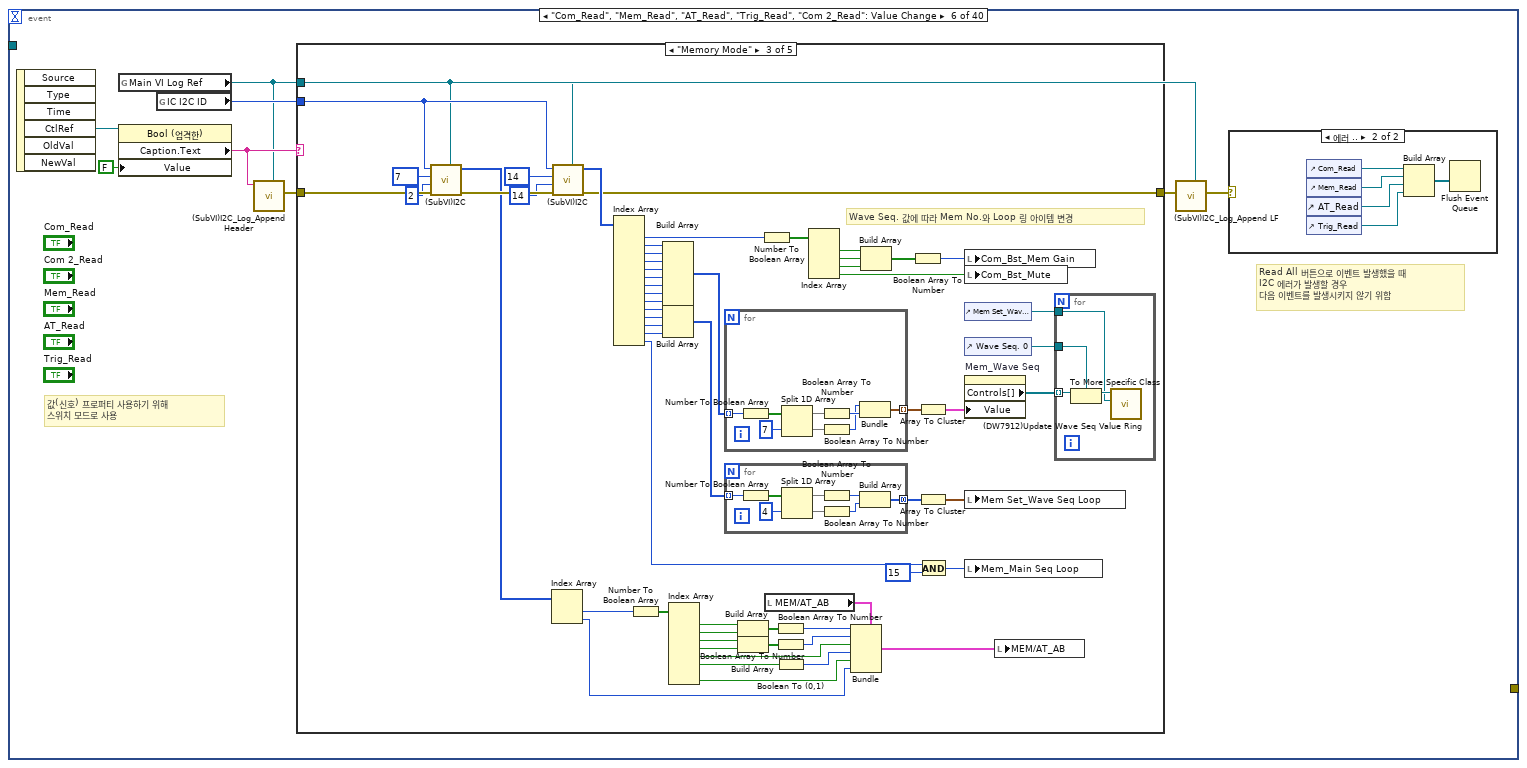
[diagram p20: hidden frame]
diagram:
  # "큐 해제해야 While 루프 종료됨"
  # "DW7802는 아직 정식 출시되지 않은 IC임\n개발2팀, FAE3팀에서 테스트하기 위해 추가된 기능이 많기 때문에\n해당 기능은 정식 출시 후에 협의하여 숨겨야 함\n(Common 2, Hidden, Fuse, Script 등)\n\nIC가 Fab out 되기 전에 개발2팀이 FPGA로 구현하여 테스트 진행했는데,\nFPGA의 몇몇 레지스터 주소가 실제 IC의 주소와 다름\n이런 레지스터는 북마크로 #7802_FPGA 라고 표기하였음\n(현재 개발2팀 요청으로 IC 레지스터로 다시 수정한 상태)"
  # "스크립트 실행을 위해 I2C Master 2의 코드를 가져옴 (GUI Log Class)"
  # "Mode Tab의 Memory Mode, Auto Track Mode 페이지에서 공용으로 사용\nTrig Mode 페이지로 이동할 때 숨겨야 함"
  # "Memory Mode일 때만 활성화,\n기본 값이 RTP Mode이므로\n초기에 비활성화함"
  # "TRIG Enable이 참일 때에만 보이는 페이지\n기본 값이 거짓이므로 초기에 숨김"
  # "8bit, 16bit 설정에 따라 16진수 자릿수 변경되도록 이벤트를 발생시킴"
  # "Trigger 그림이 그려지도록 값(신호) 프로퍼티로 이벤트를 발생시킴"
  # "마지막 설정 값 불러오기"
  # "마지막 아이템 (48kHz가 겹침) 숨기기"
  # "마지막 아이템 (빈 문자열) 숨기기"
  n1 = invoke class="VI" method="Default Vals.Reinit All"() -> (error out=w46:errorcluster)  [unwired: 3 in, 2 out]
  n2 = property on="구획" class="Pane"(error in=w46, "Origin"=T17 {"Horizontal"=0, "Vertical"=0} ("원점")) -> (error out=w41:errorcluster)  [unwired: 1 in, 1 out]
  n3 = property on="Com_Status_Select" class="Enum (엄격한)"(error in=w41, "HideLastVal"=TRUE ("Hide Last Value")) -> (error out=w33:errorcluster)  [unwired: 1 in, 1 out]
  n4 = property on="Com_PWM_Freq" class="Ring (엄격한)"(error in=w33, "HideLastVal"=TRUE ("Hide Last Value")) -> (error out=w32:errorcluster)  [unwired: 1 in, 1 out]
  n5 = disable-structure shown="비활성화" {
    disable-tunnel: [w50 w52] -> w18
    disable-tunnel: w32 -> [w47 w52]
    frame Disabled {
      n6 = property on="Com_Status_Select" class="Enum (엄격한)"(error in=w47, "Val(Sgnl)"=T18."CHIP ID" ("값(신호)")) -> (error out=w49:errorcluster)  [unwired: 1 in, 1 out]
      n7 = property on="Read All" class="Bool (엄격한)"(error in=w49, "Val(Sgnl)"=FALSE ("값(신호)")) -> (error out=w50:errorcluster)  [unwired: 1 in, 1 out]
    }
    frame Enabled {
    }
  }
  n8 = control-ref of="Trig_Gen_Setting"() -> (w20:refnum<vi>)
  n9 = control-ref of="Hidden_Register Access"() -> (w17:refnum<vi>)
  n10 = control-ref of="Fuse_Register Access"() -> (w16:refnum<vi>)
  n11 = control-ref of="Script_Path"() -> (w5:refnum<vi>)
  n12 = Build Array(w20, w17, w16, w5) -> (w19:refnum<vi>[])
  n13 = property class="Clust"(reference=w17) -> ("Controls[]"=w15:refnum<vi>[])  [unwired: 1 in, 2 out]
  n14 = property class="Clust"(reference=w16) -> ("Controls[]"=w14:refnum<vi>[])  [unwired: 1 in, 2 out]
  n15 = call "(SubVI)Control Data_Save or Load Control Value.vi"("Val(Sgnl)"=TRUE, "Common? (f)"=TRUE, "Function"=(Ctrl)Control_Data_Save_or_Load_Control_Data_Function."Load", "error in (no error)"=w18, "Control Ref"=w19) -> ("error out"=w4:errorcluster)  [unwired: 6 in]
  n16 = Build Array (concatenate)(w15, w14) -> (w13:refnum<vi>[])
  n17 = for {
    tunnel: w13 -> [w62] mode=indexing
    n18 = control-ref of="Register 1"() -> (w60:refnum<vi>)
    n19 = To More Specific Class(target class=w60, reference=w62) -> (specific class reference=w61:refnum<vi>)  [unwired: 1 in, 1 out]
    n20 = property class="Clust"(reference=w61) -> ("Controls[]"=w59:refnum<vi>[])  [unwired: 1 in, 2 out]
    n21 = Index Array(array=w59, index #1=2 ("인덱스")) -> (element #1=w54:refnum<vi>, element #2=w53:refnum<vi>)  [unwired: 1 in]
    n22 = property class="Ctl"(reference=w54) -> (reference out=w57:refnum<vi>, "Value"=w56:variant)  [unwired: 1 in, 1 out]
    n23 = property class="Ctl"(reference=w53, "Value"=u16 0) -> ()  [unwired: 1 in, 2 out]
    n24 = property class="Ctl"(reference=w57, "Val(Sgnl)"=w56) -> ()  [unwired: 1 in, 2 out]
  }
  n25 = property on="Script_Path" class="Clust (엄격한)"(error in=w4) -> (error out=w3:errorcluster, "Value"=w2:T13)  [unwired: 1 in, 1 out]
  n26 = property on="Script_Path" class="Clust (엄격한)"(error in=w3, "Val(Sgnl)"=w2) -> (error out=w1:errorcluster)  [unwired: 1 in, 1 out]
  n27 = global read "(Var)System Variables.vi" "Haptic IC"() -> (w39:refnum<class "Haptic IC.lvclass">)
  n28 = control-ref of="Com_PWM_Freq"() -> (w38:refnum<vi>)
  n29 = control-ref of="Com_VD Clamp"() -> (w37:refnum<vi>)
  n30 = control-ref of="Com_Mode_Play Mode"() -> (w30:refnum<vi>)
  n31 = property class="Haptic IC.lvclass"(reference=w39, error in=w1, "Accessors:freq ref"=w38, "Accessors:voltage range ref"=w37, "Accessors:mode ref"=w30) -> (reference out=w36:refnum<class "Haptic IC.lvclass">, error out=w23:errorcluster)
  n32 = global write "(Var)System Variables.vi" "Haptic IC"(w36) -> ()
  n33 = property on="Mode Tab" class="TabCtl (엄격한)"() -> ("Pages"=w24:refnum<vi>[])  [unwired: 2 in, 2 out]
  n34 = Index Array(array=w24, index=2 ("인덱스")) -> (element=w25:refnum<vi>)
  n35 = property class="Page"(reference=w25, error in=w23, "PageVis"=FALSE ("페이지 보이기")) -> (error out=w22:errorcluster)  [unwired: 1 out]
  n36 = call "line limit fgv.vi"("function"=line_limit_fgv_enum."Write", "line limit in"=1000) -> ("error out"=w10:errorcluster)  [unwired: 8 in, 1 out]
  n37 = property on="Com_PWM_Mode" class="Ring (엄격한)"(error in=w22, "DisabledEnum"=T15."Disabled and Grayed Out" ("비활성화")) -> (error out=w29:errorcluster)  [unwired: 1 in, 1 out]
  n38 = global read "(Var)System Variables.vi" "Main VI Log Ref"() -> (w8:refnum<vi>)
  n39 = property on="MEM/AT_AB" class="Clust (엄격한)"(error in=w29, "Visible"=TRUE ("보이기")) -> (error out=w28:errorcluster)  [unwired: 1 in, 1 out]
  n40 = call "create new obj.vi"("error in (no error)"=w10, "log ref"=w8) -> ("error out"=w9:errorcluster, "GUI Log Class.lvclass"=w7:refnum<class "GUI Log Class.lvclass">)  [unwired: 8 in]
  n41 = while {
    tunnel: [w66] -> w44
    tunnel: w28 -> [_]
    tunnel: w9 -> [_]
    tunnel: w7 -> [w63]
    tunnel: [w63] -> w6
    stop <- w65 stop-if-true
    n42 = event shown="[19] \"Hidden_Register Access.Register 1.R Btn\", \"Hidden_Register Access.Register 2.R Btn\", \"Hidden_Register Access.Register 3.R Btn\", \"Hidden_Register Access.Register 4.R Btn\", \"Hidden_Register Access.Register 5.R Btn\", \"Hidden_Register Access.Register 6.R Btn\", \"Hidden_Register Access.Register 7.R Btn\", \"Hidden_Register Access.Register 8.R Btn\", \"Hidden_Register Access.Register 9.R Btn\", \"Hidden_Register Access.Register 10.R Btn\", \"Hidden_Register Access.Register 11.R Btn\", \"Hidden_Register Access.Register 12.R Btn\", \"Hidden_Register Access.Register 13.R Btn\", \"Hidden_Register Access.Register 14.R Btn\", \"Hidden_Register Access.Register 15.R Btn\", \"Hidden_Register Access.Register 16.R Btn\", \"Hidden_Register Access.Register 17.R Btn\", \"Hidden_Register Access.Register 18.R Btn\", \"Hidden_Register Access.Register 19.R Btn\", \"Hidden_Register Access.Register 20.R Btn\", \"Hidden_Register Access.Register 21.R Btn\", \"Hidden_Register Access.Register 22.R Btn\", \"Hidden_Register Access.Register 23.R Btn\", \"Hidden_Register Access.Register 24.R Btn\", \"Fuse_Register Access.Register 1.R Btn\", \"Fuse_Register Access.Register 2.R Btn\", \"Fuse_Register Access.Register 3.R Btn\", \"Fuse_Register Access.Register 4.R Btn\", \"Fuse_Register Access.Register 5.R Btn\", \"Fuse_Register Access.Register 6.R Btn\", \"Fuse_Register Access.Register 7.R Btn\", \"Fuse_Register Access.Register 8.R Btn\", \"Fuse_Register Access.Register 9.R Btn\", \"Fuse_Register Access.Register 10.R Btn\", \"Fuse_Register Access.Register 11.R Btn\", \"Fuse_Register Access.Register 12.R Btn\", \"Fuse_Register Access.Register 13.R Btn\", \"Fuse_Register Access.Register 14.R Btn\", \"Fuse_Register Access.Register 15.R Btn\", \"Fuse_Register Access.Register 16.R Btn\", \"Fuse_Register Access.Register 17.R Btn\", \"Fuse_Register Access.Register 18.R Btn\", \"Fuse_Register Access.Register 19.R Btn\", \"Fuse_Register Access.Register 20.R Btn\", \"Fuse_Register Access.Register 21.R Btn\", \"Fuse_Register Access.Register 22.R Btn\", \"Fuse_Register Access.Register 23.R Btn\", \"Fuse_Register Access.Register 24.R Btn\": 값 변경" {
      selector: _ -> [_ _ _ _ _ _ _ _ _ _ _ _ _ _ _ _ _ _ _ _ _ _ _ _ _ _ _ _ _ _ _ _ _ _ _ _ _ _ _ _]
      dyn-events: _ -> [_ _ _ _ _ _ _ _ _ _ _ _ _ _ _ _ _ _ _ _ _ _ _ _ _ _ _ _ _ _ _ _ _ _ _ _ _ _ _ _]
      timeout: 100 -> [_ _ _ _ _ _ _ _ _ _ _ _ _ _ _ _ _ _ _ _ _ _ _ _ _ _ _ _ _ _ _ _ _ _ _ _ _ _ _ _]
      tunnel: [errorcluster {"status"=FALSE, "code"=0, "source"=""} ("에러 상수") _ _ _ _ _ _ _ _ _ _ _ _ _ _ _ _ _ _ _ _ _ _ _ _ _ _ _ _ _ _ _ _ _ _ _ _ _ _ _] -> w66
      tunnel: w63 -> [_ _ _ _ _ _ _ _ _ _ _ _ _ _ _ _ _ _ _ _ _ _ _ w820 _ _ _ _ _ _ _ _ _ _ _ _ _ _ _ _]
      event Timeout {
        n43 = event-data() -> ()  [unwired: 1 in, 3 out]
      }
      event "Mode Tab": Value Change {
        n44 = event-data() -> ("NewVal"=w71:T2)  [unwired: 1 in, 5 out]
        n45 = case shown="\"Memory Mode\", \"Auto Track Mode\"" w71 {
          tunnel: [FALSE TRUE] -> w70
          frame Default {
          }
          frame "Memory Mode", "Auto Track Mode" {
          }
        }
        n46 = property on="MEM/AT_AB" class="Clust (엄격한)"("Visible"=w70) -> ()  [unwired: 2 in, 2 out]
      }
      event "Com_Status_Select": Value Change {
        n47 = event-data() -> ()  [unwired: 1 in, 6 out]
        n48 = global read "(Var)System Variables.vi" "Main VI Log Ref"() -> (w75:refnum<vi>)
        n49 = global read "(Var)System Variables.vi" "IC I2C ID"() -> (w78:u8)
        n50 = Format Into String("Com_Status_Select") -> (resulting string=w77:string)  [unwired: 3 in, 1 out]
        n51 = call "(SubVI)I2C_Log_Append Header.vi"("Log Ref"=w75, "Header"=w77) -> ("error out"=w79:errorcluster)  [unwired: 9 in]
        n52 = case shown="\"BEMF Status\"" "Com_Status_Select" {
          tunnel: [w85 w97 w105 w122 w149 w160 w171 w183 w196] -> w80
          tunnel: w79 -> [w82 w92 w102 w141 w153 w164 w175 w190 w193]
          tunnel: w75 -> [w83 w93 w103 w120 w144 w155 w166 w184 w194]
          tunnel: w78 -> [w84 w94 w104 w121 w145 w156 w167 w185 w195]
          tunnel: [w81 w91 w101 w142 w143 w154 w165 w191 w192] -> w74
          frame "Chip ID", Default {
            # "현재 DW7802 Chip ID는 0x00으로 되어있음\n정식 출시 후 변경되면 수정해야 함"
            n53 = call-poly "(SubVI)I2C.vi"("Log Ref"=w83, "error in (no error)"=w82, "Address"=u8 0 ("Start Address"), "ID"=w84) -> ("error out"=w81:errorcluster, "Read Data"=w86:u8)  [unwired: 5 in, 1 out]
            n54 = call "(SubVI)Chip ID Converter.vi"("Chip ID"=w86) -> ("Chip Type"=w88:string)  [unwired: 10 in]
            n55 = Format Into String(format string=" / Info : 0x%02x" ("포맷 문자열"), initial string=w88, w86) -> (resulting string=w85:string)  [unwired: 1 in, 1 out]
          }
          frame "VBAT" {
            n56 = call-poly "(SubVI)I2C.vi"("Log Ref"=w93, "error in (no error)"=w92, "Address"=u8 9 ("Start Address"), "ID"=w94) -> ("error out"=w91:errorcluster, "Read Data"=w98:u8)  [unwired: 5 in, 1 out]
            n57 = To Unsigned Word Integer(number=w98) -> (unsigned 16bit integer=w90:u16)
            n58 = Multiply(x=w90, y=u16 24) -> (x*y=w96:u16)
            n59 = Format Into String(format string="VBAT : %dmV" ("포맷 문자열"), w96) -> (resulting string=w97:string)  [unwired: 2 in, 1 out]
          }
          frame "Status" {
            n60 = call-poly "(SubVI)I2C.vi"("Log Ref"=w103, "error in (no error)"=w102, "Address"=u8 1 ("Start Address"), "ID"=w104) -> ("error out"=w101:errorcluster, "Read Data"=w107:u8)  [unwired: 5 in, 1 out]
            n61 = case shown="1, 기본" w107 {
              selector: w107 -> [_ w117]
              tunnel: string[] ["OCP", "TSD", "UVLO", "FIFO Empty", "FIFO Full", "Act Open", "Act Short", "TRIG In"] -> [_ w115]
              tunnel: ["Return 0" ("trimmed string") w110] -> w105
              frame 0 {
              }
              frame 1, Default {
                n62 = Number To Boolean Array(number=w117) -> (Boolean array=w116:bool[])
                n63 = for {
                  tunnel: w116 -> [w118] mode=indexing
                  tunnel: w115 -> [w119] mode=indexing
                  tunnel: [w119] -> w114 mode=indexing if=w118
                }
                n64 = Array To Spreadsheet String(delimiter (Tab)=" / " ("구분 문자 (탭)"), array=w114, 3:"%s" ("포맷 문자열")) -> (spreadsheet string=w111:string)
                n65 = call <vilib>:"Trim Whitespace.vi"("string"=w111) -> ("trimmed string"=w110:string)  [unwired: 1 in]
              }
            }
          }
          frame "ACT F0 Value" {
            # "#7802_FPGA\nIC : 0x26\nFPGA : 0x42"
            n66 = call-poly "(SubVI)I2C.vi"("Log Ref"=w120, "error in (no error)"=w141, "Size to Read"=u16 2, "Start Address"=u8 38, "ID"=w121) -> ("error out"=w142:errorcluster, "Read Data"=w137:u8[])  [unwired: 4 in, 1 out]
            n67 = Index Array(array=w137) -> (element #1=w136:u8, element #2=w129:u8)  [unwired: 2 in]
            n68 = Number To Boolean Array(number=w136) -> (Boolean array=w135:bool[])
            n69 = Index Array(array=w135, index #1=7 ("인덱스"), index #2=0 ("인덱스")) -> (element #1=w125:bool, element #2=w132:bool)
            n70 = Boolean To (0,1)(Boolean=w132) -> (0, 1=w131:i16)
            n71 = To Unsigned Byte Integer(number=w131) -> (unsigned 8bit integer=w130:u8)
            n72 = Join Numbers(hi=w130, lo=w129) -> ((hi.lo)=w128:u16)
            n73 = Format Into String(format string="Value : %d" ("포맷 문자열"), w128) -> (resulting string=w123:string)  [unwired: 2 in, 1 out]
            n74 = Select(t="ACT F0 Freq. Error / ", s=w125, f="") -> (s? t:f=w124:string)
            n75 = Concatenate Strings(w124, w123) -> (w122:string)
          }
          frame "FIFO Status" {
            n76 = call-poly "(SubVI)I2C.vi"("Log Ref"=w144, "error in (no error)"=w153, "Size to Read"=u16 2, "Start Address"=u8 49, "ID"=w145) -> ("error out"=w143:errorcluster, "Read Data"=w150:u8[])  [unwired: 4 in, 1 out]
            n77 = Type Cast(type=u16 0 ("타입"), x=w150) -> (*(type *) &x=w147:u16)
            n78 = Format Into String(format string="Value : %d" ("포맷 문자열"), w147) -> (resulting string=w149:string)  [unwired: 2 in, 1 out]
          }
          frame "FIFO Full Level" {
            n79 = call-poly "(SubVI)I2C.vi"("Log Ref"=w155, "error in (no error)"=w164, "Size to Read"=u16 2, "Start Address"=u8 45, "ID"=w156) -> ("error out"=w154:errorcluster, "Read Data"=w161:u8[])  [unwired: 4 in, 1 out]
            n80 = Type Cast(type=u16 0 ("타입"), x=w161) -> (*(type *) &x=w158:u16)
            n81 = Format Into String(format string="FIFO Full Value : %d Byte" ("포맷 문자열"), w158) -> (resulting string=w160:string)  [unwired: 2 in, 1 out]
          }
          frame "FIFO Empty Level" {
            n82 = call-poly "(SubVI)I2C.vi"("Log Ref"=w166, "error in (no error)"=w175, "Size to Read"=u16 2, "Start Address"=u8 47, "ID"=w167) -> ("error out"=w165:errorcluster, "Read Data"=w172:u8[])  [unwired: 4 in, 1 out]
            n83 = Type Cast(type=u16 0 ("타입"), x=w172) -> (*(type *) &x=w169:u16)
            n84 = Format Into String(format string="FIFO Empty Value : %d Byte" ("포맷 문자열"), w169) -> (resulting string=w171:string)  [unwired: 2 in, 1 out]
          }
          frame "ACT Resistance" {
            n85 = call-poly "(SubVI)I2C.vi"("Log Ref"=w184, "error in (no error)"=w190, "Size to Read"=u16 2, "Start Address"=u8 51, "ID"=w185) -> ("error out"=w191:errorcluster, "Read Data"=w186:u8[])  [unwired: 4 in, 1 out]
            n86 = Index Array(array=w186) -> (element #1=w182:u8, element #2=w181:u8)  [unwired: 2 in]
            n87 = And(x=w181, y=u8 15) -> (x .and. y?=w177:u8)
            n88 = Multiply(x=w177, y=0.0625) -> (x*y=w179:dbl)
            n89 = Add(x=w182, y=w179) -> (x+y=w178:dbl)
            n90 = Format Into String(format string="Resistance : %#g" ("포맷 문자열"), w178) -> (resulting string=w183:string)  [unwired: 2 in, 1 out]
          }
          frame "BEMF Status" {
            # "#7802_FPGA\nIC : 0x35\nFPGA : 0x55"
            n91 = call-poly "(SubVI)I2C.vi"("Log Ref"=w194, "error in (no error)"=w193, "Address"=u8 53 ("Start Address"), "ID"=w195) -> ("error out"=w192:errorcluster, "Read Data"=w198:u8)  [unwired: 5 in, 1 out]
            n92 = case shown="1, 기본" w198 {
              selector: w198 -> [_ w208]
              tunnel: string[] ["BEMF Low", "BEMF High"] -> [_ w206]
              tunnel: ["Return 0" ("trimmed string") w201] -> w196
              frame 0 {
              }
              frame 1, Default {
                n93 = Number To Boolean Array(number=w208) -> (Boolean array=w207:bool[])
                n94 = for {
                  tunnel: w207 -> [w209] mode=indexing
                  tunnel: w206 -> [w210] mode=indexing
                  tunnel: [w210] -> w205 mode=indexing if=w209
                }
                n95 = Array To Spreadsheet String(delimiter (Tab)=" / " ("구분 문자 (탭)"), array=w205, 3:"%s" ("포맷 문자열")) -> (spreadsheet string=w202:string)
                n96 = call <vilib>:"Trim Whitespace.vi"("string"=w202) -> ("trimmed string"=w201:string)  [unwired: 1 in]
              }
            }
          }
        }
        "Com_Status_Result" <- w80
        n97 = call "(SubVI)I2C_Log_Append LF.vi"("Log Ref"=w75, "error in (no error)"=w74) -> ()  [unwired: 9 in, 1 out]
      }
      event "Com_Status_Select": Operate Menu Activation; "Com_Status_Select": event #0x43 {
        # "현재 아이템과 동일한 아이템을 다시 선택해도\n값 변경 이벤트가 발생하도록\n열거형 클릭 시 임시로 값을 변경함\n\n값을 변경하지 않고 메뉴 해제 시 기존 값으로 다시 변경"
        n98 = event-data() -> ("CtlRef"=w216:refnum<vi>)  [unwired: 1 in, 3 out]
        n99 = property class="Enum (엄격한)"(reference=w216) -> (reference out=w213:refnum<vi>, error out=w214:errorcluster, "Value"=w215:T8)  [unwired: 1 in]
        n100 = feedback #1() -> (w211:T8)  [unwired: 1 in]
        n101 = case shown="\"Chip ID\", 기본" w215 {
          tunnel: w214 -> [w219 w222]
          tunnel: w213 -> [w220 w223]
          tunnel: [w218 w221] -> w212
          tunnel: w211 -> [_ w221]
          frame "Chip ID", Default {
            # "열거형 클릭 시 임시로 빈 문자열 아이템으로 변경,\n기존 값은 피드백 노드에 저장"
            n102 = property class="Enum (엄격한)"(reference=w220, error in=w219, "Value"=T8."" ("값")) -> ("Value"=w218:T8)  [unwired: 2 out]
          }
          frame "" {
            # "열거형 메뉴 해제 시 기존 값으로 다시 변경"
            n103 = property class="Enum (엄격한)"(reference=w223, error in=w222, "Value"=w221) -> ()  [unwired: 2 out]
          }
        }
        n104 = feedback-in #1(w212) -> ()
      }
      event "Read All": Value Change {
        w224 = FALSE ("값(신호)")
        # "Read All 버튼은 현재 사용하지 않음"
        # "값(신호) 프로퍼티 사용하기 위해\n스위치 모드로 사용"
        n105 = event-data() -> ()  [unwired: 1 in, 6 out]
        n106 = local write "Read All"(FALSE ("Read All")) -> ()
        n107 = property on="Com_Read" class="Bool (엄격한)"("Val(Sgnl)"=w224) -> (error out=w228:errorcluster)  [unwired: 2 in, 1 out]
        n108 = property on="Mem_Read" class="Bool (엄격한)"(error in=w228, "Val(Sgnl)"=w224) -> (error out=w226:errorcluster)  [unwired: 1 in, 1 out]
        n109 = property on="AT_Read" class="Bool (엄격한)"(error in=w226, "Val(Sgnl)"=w224) -> (error out=w225:errorcluster)  [unwired: 1 in, 1 out]
        n110 = property on="Trig_Read" class="Bool (엄격한)"(error in=w225, "Val(Sgnl)"=w224) -> ()  [unwired: 1 in, 2 out]
      }
      event "Com_Read", "Mem_Read", "AT_Read", "Trig_Read", "Com 2_Read": Value Change {
        # "Read All 버튼으로 이벤트 발생했을 때\nI2C 에러가 발생할 경우 \n다음 이벤트를 발생시키지 않기 위함"
        # "값(신호) 프로퍼티 사용하기 위해\n스위치 모드로 사용"
        n111 = event-data() -> ("CtlRef"=w236:refnum<vi>)  [unwired: 1 in, 5 out]
        n112 = global read "(Var)System Variables.vi" "Main VI Log Ref"() -> (w230:refnum<vi>)
        n113 = property class="Bool (엄격한)"(reference=w236, "Value"=FALSE ("값")) -> ("Caption.Text"=w233:string)  [unwired: 1 in, 2 out]
        n114 = global read "(Var)System Variables.vi" "IC I2C ID"() -> (w232:u8)
        n115 = call "(SubVI)I2C_Log_Append Header.vi"("Log Ref"=w230, "Header"=w233) -> ("error out"=w234:errorcluster)  [unwired: 9 in]
        n116 = case shown="\"Memory Mode\"" w233 {
          tunnel: [w281 w288 w408 w522 w564] -> w231
          tunnel: w234 -> [w272 w289 w440 w508 w552]
          tunnel: w230 -> [w271 w287 w426 w473 w550]
          tunnel: w232 -> [w270 w286 w427 w474 w551]
          frame "Common", Default {
            n117 = disable-structure shown="활성화" {
              disable-tunnel: [T19[] [{"Address"=11, "Delay(ms)"=0}, {"Address"=2, "Delay(ms)"=0}, {"Address"=5, "Delay(ms)"=0}, {"Address"=10, "Delay(ms)"=0}, {"Address"=35, "Delay(ms)"=0}, {"Address"=36, "Delay(ms)"=0}, {"Address"=37, "Delay(ms)"=0}] ("Address to Read") T19[] [{"Address"=11, "Delay(ms)"=0}, {"Address"=2, "Delay(ms)"=0}, {"Address"=5, "Delay(ms)"=0}, {"Address"=10, "Delay(ms)"=0}, {"Address"=35, "Delay(ms)"=0}, {"Address"=63, "Delay(ms)"=0}, {"Address"=64, "Delay(ms)"=0}] ("Address to Read")] -> w280
              frame Enabled {
                # "IC"
              }
              frame Disabled {
                # "#7802_FPGA"
              }
            }
            n118 = call-poly "(SubVI)I2C.vi"("Log Ref"=w271, "error in (no error)"=w272, "Address to Read"=w280, "ID"=w270) -> ("error out"=w281:errorcluster, "Read Data"=w279:u8[])  [unwired: 5 in, 1 out]
            n119 = Index Array(array=w279) -> (element #1=w267:u8, element #2=w253:u8, element #3=w252:u8, element #4=w266:u8, element #5=w239:u8, element #6=w238:u8, element #7=w237:u8)  [unwired: 7 in]
            n120 = Number To Boolean Array(number=w253) -> (Boolean array=w265:bool[])
            n121 = Number To Boolean Array(number=w252) -> (Boolean array=w278:bool[])
            n122 = Number To Boolean Array(number=w239) -> (Boolean array=w251:bool[])
            n123 = Number To Boolean Array(number=w238) -> (Boolean array=w247:bool[])
            n124 = Index Array(array=w265) -> (element #1=w264:bool, element #2=w260:bool)  [unwired: 2 in]
            n125 = Index Array(array=w278) -> (element #1=w277:bool, element #2=w276:bool, element #3=w268:bool)  [unwired: 3 in]
            n126 = Index Array(array=w251) -> (element=w250:bool)  [unwired: 1 in]
            n127 = Index Array(array=w247, index #2=4 ("인덱스")) -> (element #1=w242:bool, element #2=w245:bool, element #3=w244:bool)  [unwired: 2 in]
            n128 = Build Array(w277, w276) -> (w275:bool[])
            n129 = Boolean To (0,1)(Boolean=w242) -> (0, 1=w249:i16)
            n130 = Build Array(w245, w244) -> (w246:bool[])
            n131 = To Unsigned Byte Integer(number=w249) -> (unsigned 8bit integer=w241:u8)
            n132 = Boolean Array To Number ("불리언 배열을 숫자로")(Boolean array=w275) -> (number=w274:u8)
            n133 = Boolean To (0,1)(Boolean=w268) -> (0, 1=w273:i16)
            n134 = Boolean Array To Number ("불리언 배열을 숫자로")(Boolean array=w246) -> (number=w243:u16)
            n135 = Join Numbers(hi=w241, lo=w237) -> ((hi.lo)=w248:u16)
            n136 = property on="Mode Tab" class="TabCtl (엄격한)"() -> (error out=w259:errorcluster, "Pages"=w263:refnum<vi>[])  [unwired: 2 in, 1 out]
            n137 = local write "Com_Mode_Play Mode"(w267) -> ()
            n138 = local write "Com_Mode_Int Enable"(w264) -> ()
            n139 = local write "Com_Mode_Trig Enable"(w260) -> ()
            n140 = local write "Com_PWM_Freq"(w274) -> ()
            n141 = local write "Com_PWM_Mode"(w273) -> ()
            n142 = local write "Com_VD Clamp"(w266) -> ()
            n143 = local write "Com_ACT_CAL F0"(w250) -> ()
            n144 = local write "Com_ACT_Freq Range"(w243) -> ()
            n145 = local write "Com_ACT_F0 In"(w248) -> ()
            n146 = case shown="1, 기본" w267 {
              tunnel: [T15."Enabled" ("비활성화") T15."Disabled and Grayed Out" ("비활성화")] -> w269
              frame 0 {
              }
              frame 1, Default {
              }
            }
            n147 = Index Array(array=w263, index=2 ("인덱스")) -> (element=w262:refnum<vi>)
            n148 = property class="Page"(reference=w262, error in=w259, "PageVis"=w260) -> (error out=w254:errorcluster)  [unwired: 1 out]
            n149 = property on="Mode Tab" class="TabCtl (엄격한)"(error in=w254) -> (error out=w255:errorcluster, "Value"=w257:T2)  [unwired: 1 in, 1 out]
            n150 = Not Equal?(x=w257, y=T2."Trig Mode") -> (x != y?=w258:bool)
            n151 = property on="Com_PWM_Mode" class="Ring (엄격한)"("DisabledEnum"=w269) -> ()  [unwired: 2 in, 2 out]
            n152 = property on="MEM/AT_AB" class="Clust (엄격한)"(error in=w255, "Visible"=w258) -> ()  [unwired: 1 in, 2 out]
          }
          frame "Common 2" {
            n153 = disable-structure shown="활성화" {
              disable-tunnel: w289 -> [w333 w383]
              disable-tunnel: [w304 w354] -> w288
              disable-tunnel: w287 -> [w291 w343]
              disable-tunnel: w286 -> [w290 w342]
              frame Enabled {
                # "IC"
                n154 = call-poly "(SubVI)I2C.vi"("Log Ref"=w291, "error in (no error)"=w333, "Address to Read"=T19[] [{"Address"=3, "Delay(ms)"=0}, {"Address"=33, "Delay(ms)"=0}, {"Address"=34, "Delay(ms)"=0}], "ID"=w290) -> ("error out"=w305:errorcluster, "Read Data"=w338:u8[])  [unwired: 5 in, 1 out]
                n155 = call-poly "(SubVI)I2C.vi"("Log Ref"=w291, "error in (no error)"=w305, "Size to Read"=u16 6, "Start Address"=u8 43, "ID"=w290) -> ("error out"=w304:errorcluster, "Read Data"=w303:u8[])  [unwired: 4 in, 1 out]
                n156 = Index Array(array=w303) -> (element #1=w302:u8, element #2=w301:u8, element #3=w300:u8, element #4=w299:u8, element #5=w298:u8, element #6=w297:u8)  [unwired: 6 in]
                n157 = Index Array(array=w338) -> (element #1=w329:u8, element #2=w331:u8, element #3=w330:u8)  [unwired: 3 in]
                n158 = Join Numbers(hi=w302, lo=w301) -> ((hi.lo)=w293:u16)
                n159 = Join Numbers(hi=w300, lo=w299) -> ((hi.lo)=w296:u16)
                n160 = Join Numbers(hi=w298, lo=w297) -> ((hi.lo)=w295:u16)
                n161 = Number To Boolean Array(number=w329) -> (Boolean array=w328:bool[])
                n162 = Number To Boolean Array(number=w331) -> (Boolean array=w332:bool[])
                n163 = Number To Boolean Array(number=w330) -> (Boolean array=w337:bool[])
                n164 = Array To Cluster(array=w328) -> (cluster=w327:T21)
                n165 = Index Array(array=w332) -> (element #1=w325:bool, element #2=w324:bool, element #3=w319:bool, element #4=w320:bool, element #5=w321:bool, element #6=w318:bool, element #7=w317:bool, element #8=w316:bool)  [unwired: 8 in]
                n166 = Index Array(array=w337) -> (element #1=w336:bool, element #2=w335:bool, element #5=w313:bool, element #6=w312:bool, element #7=w311:bool, element #8=w310:bool)  [unwired: 8 in, 2 out]
                n167 = Build Array(w325, w324, w319, w320) -> (w326:bool[])
                n168 = Build Array(w321, w318, w317, w316) -> (w322:bool[])
                n169 = Build Array(w336, w335) -> (w334:bool[])
                n170 = Build Array(w313, w312, w311, w310) -> (w314:bool[])
                n171 = Subtract(x=u16 6144, y=w293) -> (x-y=w292:u16)
                n172 = Boolean Array To Number ("불리언 배열을 숫자로")(Boolean array=w326) -> (number=w323:u8)
                n173 = Boolean Array To Number ("불리언 배열을 숫자로")(Boolean array=w322) -> (number=w315:u8)
                n174 = Boolean Array To Number ("불리언 배열을 숫자로")(Boolean array=w334) -> (number=w309:u8)
                n175 = Boolean Array To Number ("불리언 배열을 숫자로")(Boolean array=w314) -> (number=w308:u8)
                n176 = local write "Com 2_FIFO_Size"(w292) -> ()
                n177 = local write "Com 2_FIFO_Full Level"(w296) -> ()
                n178 = local write "Com 2_FIFO_Empty Level"(w295) -> ()
                n179 = local write "Com 2_INTZ"(w327) -> ()
                n180 = local write "Com 2_ZXD_GND Time"(w323) -> ()
                n181 = local write "Com 2_ZXD_Null Time"(w315) -> ()
                n182 = local write "Com 2_ZXD_Sense Time"(w309) -> ()
                n183 = local write "Com 2_ZXD_BEMF Gain"(w308) -> ()
              }
              frame Disabled {
                # "#7802_FPGA"
                n184 = call-poly "(SubVI)I2C.vi"("Log Ref"=w343, "error in (no error)"=w383, "Address to Read"=T19[] [{"Address"=3, "Delay(ms)"=0}, {"Address"=33, "Delay(ms)"=0}, {"Address"=34, "Delay(ms)"=0}, {"Address"=73, "Delay(ms)"=0}, {"Address"=74, "Delay(ms)"=0}], "ID"=w342) -> ("error out"=w355:errorcluster, "Read Data"=w388:u8[])  [unwired: 5 in, 1 out]
                n185 = call-poly "(SubVI)I2C.vi"("Log Ref"=w343, "error in (no error)"=w355, "Size to Read"=u16 4, "Start Address"=u8 45, "ID"=w342) -> ("error out"=w354:errorcluster, "Read Data"=w353:u8[])  [unwired: 4 in, 1 out]
                n186 = Index Array(array=w353) -> (element #1=w352:u8, element #2=w351:u8, element #3=w350:u8, element #4=w349:u8)  [unwired: 4 in]
                n187 = Index Array(array=w388) -> (element #1=w379:u8, element #2=w381:u8, element #3=w380:u8, element #4=w341:u8, element #5=w340:u8)  [unwired: 5 in]
                n188 = Join Numbers(hi=w352, lo=w351) -> ((hi.lo)=w348:u16)
                n189 = Join Numbers(hi=w350, lo=w349) -> ((hi.lo)=w347:u16)
                n190 = Join Numbers(hi=w341, lo=w340) -> ((hi.lo)=w345:u16)
                n191 = Number To Boolean Array(number=w379) -> (Boolean array=w378:bool[])
                n192 = Number To Boolean Array(number=w381) -> (Boolean array=w382:bool[])
                n193 = Number To Boolean Array(number=w380) -> (Boolean array=w387:bool[])
                n194 = Array To Cluster(array=w378) -> (cluster=w377:T21)
                n195 = Index Array(array=w382) -> (element #1=w375:bool, element #2=w374:bool, element #3=w369:bool, element #4=w370:bool, element #5=w371:bool, element #6=w368:bool, element #7=w367:bool, element #8=w366:bool)  [unwired: 8 in]
                n196 = Index Array(array=w387) -> (element #1=w386:bool, element #2=w385:bool, element #5=w363:bool, element #6=w362:bool, element #7=w361:bool, element #8=w360:bool)  [unwired: 8 in, 2 out]
                n197 = Build Array(w375, w374, w369, w370) -> (w376:bool[])
                n198 = Build Array(w371, w368, w367, w366) -> (w372:bool[])
                n199 = Build Array(w386, w385) -> (w384:bool[])
                n200 = Build Array(w363, w362, w361, w360) -> (w364:bool[])
                n201 = Subtract(x=u16 6144, y=w345) -> (x-y=w344:u16)
                n202 = Boolean Array To Number ("불리언 배열을 숫자로")(Boolean array=w376) -> (number=w373:u8)
                n203 = Boolean Array To Number ("불리언 배열을 숫자로")(Boolean array=w372) -> (number=w365:u8)
                n204 = Boolean Array To Number ("불리언 배열을 숫자로")(Boolean array=w384) -> (number=w359:u8)
                n205 = Boolean Array To Number ("불리언 배열을 숫자로")(Boolean array=w364) -> (number=w358:u8)
                n206 = local write "Com 2_FIFO_Full Level"(w348) -> ()
                n207 = local write "Com 2_FIFO_Empty Level"(w347) -> ()
                n208 = local write "Com 2_INTZ"(w377) -> ()
                n209 = local write "Com 2_ZXD_GND Time"(w373) -> ()
                n210 = local write "Com 2_ZXD_Null Time"(w365) -> ()
                n211 = local write "Com 2_ZXD_Sense Time"(w359) -> ()
                n212 = local write "Com 2_ZXD_BEMF Gain"(w358) -> ()
                n213 = local write "Com 2_FIFO_Size"(w344) -> ()
              }
            }
          }
          frame "Memory Mode" {
            # "Wave Seq. 값에 따라 Mem No.와 Loop 링 아이템 변경"
            n214 = call-poly "(SubVI)I2C.vi"("Log Ref"=w426, "error in (no error)"=w440, "Size to Read"=u16 2, "Start Address"=u8 7, "ID"=w427) -> ("error out"=w429:errorcluster, "Read Data"=w390:u8[])  [unwired: 4 in, 1 out]
            n215 = Index Array(array=w390) -> (element #1=w399:u8, element #2=w392:u8)  [unwired: 2 in]
            n216 = call-poly "(SubVI)I2C.vi"("Log Ref"=w426, "error in (no error)"=w429, "Size to Read"=u16 14, "Start Address"=u8 14, "ID"=w427) -> ("error out"=w408:errorcluster, "Read Data"=w425:u8[])  [unwired: 4 in, 1 out]
            n217 = Index Array(array=w425) -> (element #1=w424:u8, element #2=w423:u8, element #3=w422:u8, element #4=w421:u8, element #5=w420:u8, element #6=w419:u8, element #7=w418:u8, element #8=w417:u8, element #9=w416:u8, element #10=w415:u8, element #11=w414:u8, element #12=w413:u8, element #13=w412:u8, element #14=w411:u8)  [unwired: 14 in]
            n218 = Number To Boolean Array(number=w399) -> (Boolean array=w400:bool[])
            n219 = Build Array(w423, w422, w421, w420, w419, w418, w417, w416) -> (w409:u8[])
            n220 = Build Array(w415, w414, w413, w412) -> (w410:u8[])
            n221 = Index Array(array=w400) -> (element #1=w402:bool, element #2=w403:bool, element #3=w405:bool, element #4=w406:bool, element #5=w395:bool, element #6=w407:bool, element #8=w393:bool)  [unwired: 8 in, 1 out]
            n222 = for {
              tunnel: w409 -> [w461] mode=indexing
              tunnel: [w455] -> w446 mode=indexing
              n223 = Number To Boolean Array(number=w461) -> (Boolean array=w460:bool[])
              n224 = Split 1D Array(array=w460, index=7 ("인덱스")) -> (first subarray=w458:bool[], second subarray=w457:bool[])
              n225 = Boolean Array To Number ("불리언 배열을 숫자로")(Boolean array=w458) -> (number=w456:u8)
              n226 = Boolean Array To Number ("불리언 배열을 숫자로")(Boolean array=w457) -> (number=w454:u8)
              n227 = Bundle(w454, w456) -> (w455:cluster{u8, u8})  [unwired: 1 in]
            }
            n228 = for {
              tunnel: w410 -> [w469] mode=indexing
              tunnel: [w462] -> w445 mode=concatenating
              n229 = Number To Boolean Array(number=w469) -> (Boolean array=w468:bool[])
              n230 = Split 1D Array(array=w468, index=4 ("인덱스")) -> (first subarray=w466:bool[], second subarray=w465:bool[])
              n231 = Boolean Array To Number ("불리언 배열을 숫자로")(Boolean array=w466) -> (number=w464:u8)
              n232 = Boolean Array To Number ("불리언 배열을 숫자로")(Boolean array=w465) -> (number=w463:u8)
              n233 = Build Array(w464, w463) -> (w462:u8[])
            }
            n234 = Build Array(w402, w403) -> (w401:bool[])
            n235 = Build Array(w405, w406) -> (w404:bool[])
            n236 = Number To Boolean Array(number=w424) -> (Boolean array=w437:bool[])
            n237 = local read "MEM/AT_AB"() -> (w398:T1)
            n238 = Boolean Array To Number(Boolean array=w401) -> (number=w397:u32)
            n239 = Boolean Array To Number(Boolean array=w404) -> (number=w396:u32)
            n240 = Boolean To (0,1)(Boolean=w407) -> (0, 1=w394:i16)
            n241 = Index Array(array=w437) -> (element #1=w434:bool, element #2=w433:bool, element #3=w432:bool, element #4=w436:bool)  [unwired: 4 in]
            n242 = Bundle(cluster=w398, "OD Cycle"=w397, "OD Level"=w396, "OD Enable"=w395, "Shape"=w394, "Enable"=w393, "Gain"=w392) -> (w391:T1)
            n243 = Build Array(w434, w433, w432) -> (w435:bool[])
            n244 = Boolean Array To Number ("불리언 배열을 숫자로")(Boolean array=w435) -> (number=w431:u8)
            n245 = Array To Cluster(array=w446) -> (cluster=w443:T22)
            n246 = Array To Cluster(array=w445) -> (cluster=w444:T23)
            n247 = And(x=w411, y=u8 15) -> (x .and. y?=w447:u8)
            n248 = local write "Com_Bst_Mem Gain"(w431) -> ()
            n249 = local write "Com_Bst_Mute"(w436) -> ()
            n250 = control-ref of="Mem Set_Wave Seq Loop"() -> (w438:refnum<vi>)
            n251 = control-ref of="Wave Seq. 0"() -> (w441:refnum<vi>)
            n252 = property on="Mem_Wave Seq" class="Clust (엄격한)"("Value"=w443) -> ("Controls[]"=w442:refnum<vi>[])  [unwired: 2 in, 2 out]
            n253 = local write "Mem Set_Wave Seq Loop"(w444) -> ()
            n254 = local write "Mem_Main Seq Loop"(w447) -> ()
            n255 = local write "MEM/AT_AB"(w391) -> ()
            n256 = for {
              tunnel: w442 -> [w452] mode=indexing
              tunnel: w441 -> [w451]
              tunnel: w438 -> [w450]
              n257 = To More Specific Class(target class=w451, reference=w452) -> (specific class reference=w453:refnum<vi>)  [unwired: 1 in, 1 out]
              n258 = call "(DW7912)Update Wave Seq Value Ring.vi"("Wave Seq Loop Ref In"=w450, "Wave Seq Ref In"=w453) -> ()  [unwired: 8 in, 2 out]
            }
          }
          frame "Auto Track Mode" {
            n259 = call-poly "(SubVI)I2C.vi"("Log Ref"=w473, "error in (no error)"=w508, "Size to Read"=u16 3, "Start Address"=u8 6 ("Address"), "ID"=w474) -> ("error out"=w507:errorcluster, "Read Data"=w505:u8[])  [unwired: 4 in, 1 out]
            n260 = Index Array(array=w505) -> (element #1=w492:u8, element #2=w483:u8, element #3=w476:u8)  [unwired: 3 in]
            n261 = call-poly "(SubVI)I2C.vi"("Log Ref"=w473, "error in (no error)"=w507, "Size to Read"=u16 8, "Start Address"=u8 30, "ID"=w474) -> ("error out"=w522:errorcluster, "Read Data"=w472:u8[])  [unwired: 4 in, 1 out]
            n262 = Number To Boolean Array(number=w492) -> (Boolean array=w506:bool[])
            n263 = Number To Boolean Array(number=w483) -> (Boolean array=w484:bool[])
            n264 = Index Array(array=w472) -> (element #1=w516:u8, element #2=w514:u8, element #3=w513:u8)  [unwired: 3 in]
            n265 = Index Array(array=w506) -> (element #1=w503:bool, element #2=w502:bool, element #3=w499:bool, element #4=w498:bool, element #5=w497:bool, element #6=w495:bool)  [unwired: 8 in, 2 out]
            n266 = Index Array(array=w484) -> (element #1=w486:bool, element #2=w487:bool, element #3=w489:bool, element #4=w490:bool, element #5=w479:bool, element #6=w491:bool, element #8=w477:bool)  [unwired: 8 in, 1 out]
            n267 = Build Array(w503, w502) -> (w504:bool[])
            n268 = Build Array(w499, w498) -> (w500:bool[])
            n269 = Build Array(w486, w487) -> (w485:bool[])
            n270 = Build Array(w489, w490) -> (w488:bool[])
            n271 = local read "MEM/AT_AB"() -> (w482:T1)
            n272 = Boolean Array To Number(Boolean array=w504) -> (number=w501:u32)
            n273 = Boolean Array To Number(Boolean array=w500) -> (number=w496:u32)
            n274 = Boolean To (0,1)(Boolean=w495) -> (0, 1=w494:i16)
            n275 = Boolean Array To Number(Boolean array=w485) -> (number=w481:u32)
            n276 = Boolean Array To Number(Boolean array=w488) -> (number=w480:u32)
            n277 = Boolean To (0,1)(Boolean=w491) -> (0, 1=w478:i16)
            n278 = Number To Boolean Array(number=w516) -> (Boolean array=w520:bool[])
            n279 = Bundle(cluster=w482, "OD Cycle"=w481, "OD Level"=w480, "OD Enable"=w479, "Shape"=w478, "Enable"=w477, "Gain"=w476) -> (w475:T1)
            n280 = Index Array(array=w520, index #5=7 ("인덱스")) -> (element #1=w519:bool, element #2=w518:bool, element #3=w521:bool, element #4=w512:bool, element #5=w510:bool)  [unwired: 4 in]
            n281 = Build Array(w519, w518, w521, w512) -> (w517:bool[])
            n282 = Boolean Array To Number ("불리언 배열을 숫자로")(Boolean array=w517) -> (number=w515:u8)
            n283 = local write "AT_Track_Loop"(w515) -> ()
            n284 = local write "AT_Track_Pattern"(w510) -> ()
            n285 = local write "AT_Track_Play"(w514) -> ()
            n286 = local write "AT_Track_Idle"(w513) -> ()
            n287 = local write "AT_Track_OD Cycle"(w501) -> ()
            n288 = local write "AT_Track_OD Level"(w496) -> ()
            n289 = local write "AT_Track_OD Enable"(w497) -> ()
            n290 = local write "AT_Track_Shape"(w494) -> ()
            n291 = local write "MEM/AT_AB"(w475) -> ()
          }
          frame "Trig Mode" {
            n292 = call-poly "(SubVI)I2C.vi"("Log Ref"=w550, "error in (no error)"=w552, "Address"=u8 4, "ID"=w551) -> ("error out"=w566:errorcluster, "Read Data"=w563:u8)  [unwired: 5 in, 1 out]
            n293 = Number To Boolean Array(number=w563) -> (Boolean array=w562:bool[])
            n294 = call-poly "(SubVI)I2C.vi"("Log Ref"=w550, "error in (no error)"=w566, "Size to Read"=u16 2, "Start Address"=u8 28, "ID"=w551) -> ("error out"=w564:errorcluster, "Read Data"=w549:u8[])  [unwired: 4 in, 1 out]
            n295 = Index Array(array=w562) -> (element #1=w560:bool, element #2=w559:bool, element #3=w558:bool, element #4=w557:bool, element #5=w553:bool, element #6=w554:bool, element #8=w555:bool)  [unwired: 8 in, 1 out]
            n296 = Index Array(array=w549) -> (element #1=w548:u8, element #2=w547:u8)  [unwired: 2 in]
            n297 = Build Array(w559, w558, w557) -> (w561:bool[])
            n298 = Number To Boolean Array(number=w548) -> (Boolean array=w546:bool[])
            n299 = Number To Boolean Array(number=w547) -> (Boolean array=w545:bool[])
            n300 = Boolean Array To Number(Boolean array=w561) -> (number=w556:u32)
            n301 = Index Array(array=w546) -> (element #1=w542:bool, element #2=w541:bool, element #3=w540:bool, element #4=w539:bool, element #5=w538:bool, element #6=w537:bool, element #7=w536:bool, element #8=w544:bool)  [unwired: 8 in]
            n302 = Index Array(array=w545) -> (element #1=w535:bool, element #2=w534:bool, element #3=w533:bool, element #4=w532:bool, element #5=w531:bool, element #6=w530:bool, element #7=w529:bool, element #8=w543:bool)  [unwired: 8 in]
            n303 = local write "Trig_Ctrl_Trig Priority"(w560) -> ()
            n304 = local write "Trig_Ctrl_Interval"(w556) -> ()
            n305 = local write "Trig_Ctrl_Trig Level"(w553) -> ()
            n306 = local write "Trig_Ctrl_Tirg Mode"(w554) -> ()
            n307 = local write "Trig_Ctrl_Restart Enable"(w555) -> ()
            n308 = Build Array(w542, w541, w540, w539, w538, w537, w536) -> (w528:bool[])
            n309 = Build Array(w535, w534, w533, w532, w531, w530, w529) -> (w526:bool[])
            n310 = Boolean Array To Number(Boolean array=w528) -> (number=w527:u32)
            n311 = Boolean Array To Number(Boolean array=w526) -> (number=w525:u32)
            n312 = Not(x=w543) -> (.not. x?=w523:bool)
            n313 = Not(x=w544) -> (.not. x?=w524:bool)
            n314 = local write "Trig_Wave_R"(w527) -> ()
            n315 = local write "Trig_Wave_R_Enable"(w524) -> ()
            n316 = local write "Trig_Wave_F"(w525) -> ()
            n317 = local write "Trig_Wave_F_Enable"(w523) -> ()
          }
        }
        n318 = call "(SubVI)I2C_Log_Append LF.vi"("Log Ref"=w230, "error in (no error)"=w231) -> ("error out"=w229:errorcluster)  [unwired: 9 in]
        n319 = case shown="에러 .." w229 {
          frame No Error {
          }
          frame Error {
            n320 = control-ref of="Com_Read"() -> (w572:refnum<vi>)
            n321 = control-ref of="Mem_Read"() -> (w571:refnum<vi>)
            n322 = control-ref of="AT_Read"() -> (w569:refnum<vi>)
            n323 = control-ref of="Trig_Read"() -> (w570:refnum<vi>)
            n324 = Build Array(w572, w571, w569, w570) -> (w573:refnum<vi>[])
            n325 = Flush Event Queue(2:w573) -> ()  [unwired: 5 in, 3 out]
          }
        }
      }
      event "Com_Mode_Play Mode": Value Change {
        n326 = event-data() -> ()  [unwired: 1 in, 6 out]
        n327 = global read "(Var)System Variables.vi" "Main VI Log Ref"() -> (w577:refnum<vi>)
        n328 = global read "(Var)System Variables.vi" "IC I2C ID"() -> (w578:u8)
        n329 = call-poly "(SubVI)I2C.vi"("Log Ref"=w577, "Data to Write"="Com_Mode_Play Mode", "Address"=u8 11, "ID"=w578) -> ()  [unwired: 6 in, 2 out]
        n330 = case shown="1, 기본" "Com_Mode_Play Mode" {
          tunnel: [T15."Enabled" ("비활성화") T15."Disabled and Grayed Out" ("비활성화")] -> w575
          frame 0 {
          }
          frame 1, Default {
          }
        }
        n331 = property on="Com_PWM_Mode" class="Ring (엄격한)"("DisabledEnum"=w575) -> ()  [unwired: 2 in, 2 out]
      }
      event "Com_Mode_Trig Enable", "Com_Mode_Int Enable": Value Change {
        n332 = event-data() -> ("CtlRef"=w581:refnum<vi>, "NewVal"=w582:bool)  [unwired: 1 in, 4 out]
        n333 = flat-sequence {
          tunnel: w582 -> [w584]
          tunnel: w581 -> [w583]
          frame #0 {
            # "Trig Enable과 Int Enable 중 하나만 사용 가능함"
            n334 = case shown="참" w584 {
              tunnel: w583 -> [_ w586]
              frame False {
              }
              frame True {
                n335 = control-ref of="Com_Mode_Trig Enable"() -> (w587:refnum<vi>)
                n336 = control-ref of="Com_Mode_Int Enable"() -> (w588:refnum<vi>)
                n337 = Build Array(w587, w588) -> (w589:refnum<vi>[])
                n338 = call "Search Unsorted 1D Array.vim"("element"=w586, "unsorted 1D array"=w589) -> ("index of element"=w585:i32)  [unwired: 9 in]
                n339 = case shown="0" w585 {
                  frame -1, Default {
                  }
                  frame 0 {
                    n340 = local write "Com_Mode_Int Enable"(FALSE ("Com_Mode_Int Enable")) -> ()
                  }
                  frame 1 {
                    n341 = local write "Com_Mode_Trig Enable"(FALSE ("Com_Mode_Int Enable")) -> ()
                  }
                }
              }
            }
          }
          frame #1 {
            n342 = Boolean To (0,1)(Boolean="Com_Mode_Int Enable") -> (0, 1=w602:i16)
            n343 = Boolean To (0,1)(Boolean="Com_Mode_Trig Enable") -> (0, 1=w599:i16)
            n344 = property on="Mode Tab" class="TabCtl (엄격한)"() -> (error out=w608:errorcluster, "Pages"=w605:refnum<vi>[])  [unwired: 2 in, 1 out]
            n345 = To Unsigned Byte Integer(number=w602) -> (unsigned 8bit integer=w604:u8)
            n346 = To Unsigned Byte Integer(number=w599) -> (unsigned 8bit integer=w600:u8)
            n347 = Logical Shift(y=i16 1, x=w600) -> (x << y=w598:u8)
            n348 = Index Array(array=w605, index=2 ("인덱스")) -> (element=w606:refnum<vi>)
            n349 = global read "(Var)System Variables.vi" "Main VI Log Ref"() -> (w597:refnum<vi>)
            n350 = Or(x=w604, y=w598) -> (x .or. y?=w601:u8)
            n351 = property class="Page"(reference=w606, error in=w608, "PageVis"="Com_Mode_Trig Enable") -> (error out=w609:errorcluster)  [unwired: 1 out]
            n352 = global read "(Var)System Variables.vi" "IC I2C ID"() -> (w596:u8)
            n353 = property on="Mode Tab" class="TabCtl (엄격한)"(error in=w609) -> (error out=w610:errorcluster, "Value"=w612:T2)  [unwired: 1 in, 1 out]
            n354 = call-poly "(SubVI)I2C.vi"("Log Ref"=w597, "Data to Write"=w601, "Address"=u8 2, "ID"=w596) -> ()  [unwired: 6 in, 2 out]
            n355 = Not Equal?(x=w612, y=T2."Trig Mode") -> (x != y?=w611:bool)
            n356 = property on="MEM/AT_AB" class="Clust (엄격한)"(error in=w610, "Visible"=w611) -> ()  [unwired: 1 in, 2 out]
          }
        }
      }
      event "Com_PWM_Freq", "Com_PWM_Mode": Value Change {
        # "Waveform Editor에서도 변경되도록 함"
        n357 = event-data() -> ()  [unwired: 1 in, 6 out]
        n358 = Logical Shift(y=i16 2, x="Com_PWM_Mode") -> (x << y=w617:u8)
        n359 = call "(SubVI)Waveform Editor_Update Sampling Rate Value.vi"("Action"=(Ctrl)Waveform_Editor_Update_Sampling_Rate_Value."Update", "Value"="Com_PWM_Freq") -> ()  [unwired: 9 in, 1 out]
        n360 = global read "(Var)System Variables.vi" "Main VI Log Ref"() -> (w620:refnum<vi>)
        n361 = Compound Arithmetic op=OR("Com_PWM_Freq", w617) -> (w616:u8)
        n362 = global read "(Var)System Variables.vi" "IC I2C ID"() -> (w621:u8)
        n363 = call-poly "(SubVI)I2C.vi"("Log Ref"=w620, "Data to Write"=w616, "Address"=u8 5, "ID"=w621) -> ()  [unwired: 6 in, 2 out]
      }
      event "Com_VD Clamp": Value Change {
        n364 = event-data() -> ()  [unwired: 1 in, 6 out]
        n365 = global read "(Var)System Variables.vi" "Main VI Log Ref"() -> (w624:refnum<vi>)
        n366 = global read "(Var)System Variables.vi" "IC I2C ID"() -> (w625:u8)
        n367 = call-poly "(SubVI)I2C.vi"("Log Ref"=w624, "Data to Write"="Com_VD Clamp", "Address"=u8 10, "ID"=w625) -> ()  [unwired: 6 in, 2 out]
      }
      event "Com_Bst_Mem Gain", "Com_Bst_Mute": Value Change {
        n368 = event-data() -> ()  [unwired: 1 in, 6 out]
        n369 = Boolean To (0,1)(Boolean="Com_Bst_Mute") -> (0, 1=w630:i16)
        n370 = To Unsigned Byte Integer(number=w630) -> (unsigned 8bit integer=w629:u8)
        n371 = Logical Shift(y=i16 3, x=w629) -> (x << y=w632:u8)
        n372 = global read "(Var)System Variables.vi" "Main VI Log Ref"() -> (w634:refnum<vi>)
        n373 = Or(x="Com_Bst_Mem Gain", y=w632) -> (x .or. y?=w626:u8)
        n374 = global read "(Var)System Variables.vi" "IC I2C ID"() -> (w635:u8)
        n375 = call-poly "(SubVI)I2C.vi"("Log Ref"=w634, "Data to Write"=w626, "Address"=u8 14, "ID"=w635) -> ()  [unwired: 6 in, 2 out]
      }
      event "Com 2_INTZ": Value Change {
        n376 = event-data() -> ()  [unwired: 1 in, 6 out]
        n377 = Cluster To Array(cluster="Com 2_INTZ") -> (array=w637:bool[])
        n378 = Boolean Array To Number ("불리언 배열을 숫자로")(Boolean array=w637) -> (number=w636:u8)
        n379 = global read "(Var)System Variables.vi" "Main VI Log Ref"() -> (w640:refnum<vi>)
        n380 = global read "(Var)System Variables.vi" "IC I2C ID"() -> (w641:u8)
        n381 = call-poly "(SubVI)I2C.vi"("Log Ref"=w640, "Data to Write"=w636, "Address"=u8 3, "ID"=w641) -> ()  [unwired: 6 in, 2 out]
      }
      event "Com 2_ZXD_Null Time", "Com 2_ZXD_GND Time": Value Change {
        n382 = event-data() -> ()  [unwired: 1 in, 6 out]
        n383 = Logical Shift(y=i16 4, x="Com 2_ZXD_Null Time") -> (x << y=w646:u8)
        n384 = global read "(Var)System Variables.vi" "Main VI Log Ref"() -> (w648:refnum<vi>)
        n385 = Or(x="Com 2_ZXD_GND Time", y=w646) -> (x .or. y?=w644:u8)
        n386 = global read "(Var)System Variables.vi" "IC I2C ID"() -> (w649:u8)
        n387 = call-poly "(SubVI)I2C.vi"("Log Ref"=w648, "Data to Write"=w644, "Address"=u8 33, "ID"=w649) -> ()  [unwired: 6 in, 2 out]
      }
      event "Com 2_ZXD_BEMF Gain", "Com 2_ZXD_Sense Time": Value Change {
        n388 = event-data() -> ()  [unwired: 1 in, 6 out]
        n389 = Logical Shift(y=i16 4, x="Com 2_ZXD_BEMF Gain") -> (x << y=w654:u8)
        n390 = global read "(Var)System Variables.vi" "Main VI Log Ref"() -> (w656:refnum<vi>)
        n391 = Or(x="Com 2_ZXD_Sense Time", y=w654) -> (x .or. y?=w652:u8)
        n392 = global read "(Var)System Variables.vi" "IC I2C ID"() -> (w657:u8)
        n393 = call-poly "(SubVI)I2C.vi"("Log Ref"=w656, "Data to Write"=w652, "Address"=u8 34, "ID"=w657) -> ()  [unwired: 6 in, 2 out]
      }
      event "Com 2_FIFO_Size": Value Change {
        w662 = u8[] []  # U8
        # "UI에서는 FIFO Size이지만 \n레지스터는 FIFO의 시작 주소이므로\nRAM Size - FIFO Size를 입력"
        # "#7802_FPGA\nIC : 0x2B\nFPGA : 0x49"
        n394 = event-data() -> ()  [unwired: 1 in, 6 out]
        n395 = Subtract(x=u16 6144, y="Com 2_FIFO_Size") -> (x-y=w659:u16)
        n396 = global read "(Var)System Variables.vi" "Main VI Log Ref"() -> (w664:refnum<vi>)
        n397 = global read "(Var)System Variables.vi" "IC I2C ID"() -> (w665:u8)
        n398 = Type Cast(type=w662, x=w659) -> (*(type *) &x=w661:u8[])
        n399 = call-poly "(SubVI)I2C.vi"("Log Ref"=w664, "Data to Write"=w661, "Start Address"=u8 43 ("Address"), "ID"=w665) -> ()  [unwired: 6 in, 2 out]
      }
      event "Com 2_FIFO_Full Level": Value Change {
        w668 = u8[] []  # U8
        n400 = event-data() -> ()  [unwired: 1 in, 6 out]
        n401 = global read "(Var)System Variables.vi" "Main VI Log Ref"() -> (w670:refnum<vi>)
        n402 = global read "(Var)System Variables.vi" "IC I2C ID"() -> (w671:u8)
        n403 = Type Cast(type=w668, x="Com 2_FIFO_Full Level") -> (*(type *) &x=w667:u8[])
        n404 = call-poly "(SubVI)I2C.vi"("Log Ref"=w670, "Data to Write"=w667, "Start Address"=u8 45 ("Address"), "ID"=w671) -> ()  [unwired: 6 in, 2 out]
      }
      event "Com 2_FIFO_Empty Level": Value Change {
        w674 = u8[] []  # U8
        n405 = event-data() -> ()  [unwired: 1 in, 6 out]
        n406 = global read "(Var)System Variables.vi" "Main VI Log Ref"() -> (w676:refnum<vi>)
        n407 = global read "(Var)System Variables.vi" "IC I2C ID"() -> (w677:u8)
        n408 = Type Cast(type=w674, x="Com 2_FIFO_Empty Level") -> (*(type *) &x=w673:u8[])
        n409 = call-poly "(SubVI)I2C.vi"("Log Ref"=w676, "Data to Write"=w673, "Start Address"=u8 47 ("Address"), "ID"=w677) -> ()  [unwired: 6 in, 2 out]
      }
      event "Com 2_Reset_SWRST": Value Change {
        # "하나씩 초기화되는 것 방지와\n초기화 속도 향상을 위해 \n패널 업데이트 연기 프로퍼티를 사용"
        # "Hidden, Fuse, Script 및 Trig_Gen의 경우\n기본 값으로 초기화하면 안되기 때문에 \nVI의 인보크 노드로 전체를 초기화하지 않고\n개별 컨트롤 초기화함"
        # "#7802_FPGA\nIC : 0x36\nFPGA : 0x5F"
        n410 = event-data() -> ()  [unwired: 1 in, 6 out]
        n411 = property on="Mode Tab" class="TabCtl (엄격한)" props=["Value", "Pages"]() -> ("Pages"=w734:refnum<vi>[])  [unwired: 2 in, 3 out]
        n412 = Boolean To (0,1)(Boolean="Com 2_Reset_SWRST") -> (0, 1=w737:i16)
        n413 = Index Array(array=w734, index=2 ("인덱스")) -> (element=w733:refnum<vi>)
        n414 = To Unsigned Byte Integer(number=w737) -> (unsigned 8bit integer=w736:u8)
        n415 = property class="Page"(reference=w733, "PageVis"=FALSE ("페이지 보이기")) -> (error out=w731:errorcluster)  [unwired: 1 in, 1 out]
        n416 = global read "(Var)System Variables.vi" "Main VI Log Ref"() -> (w740:refnum<vi>)
        n417 = global read "(Var)System Variables.vi" "IC I2C ID"() -> (w741:u8)
        n418 = property on="Com_PWM_Mode" class="Ring (엄격한)"("DisabledEnum"=T15."Disabled and Grayed Out" ("비활성화")) -> ()  [unwired: 2 in, 2 out]
        n419 = property on="MEM/AT_AB" class="Clust (엄격한)"(error in=w731, "Visible"=TRUE ("보이기")) -> ()  [unwired: 1 in, 2 out]
        n420 = call-poly "(SubVI)I2C.vi"("Log Ref"=w740, "Data to Write"=w736, "Address"=u8 54, "ID"=w741) -> ()  [unwired: 6 in, 2 out]
        n421 = control-ref of="Com 2_INTZ"() -> (w719:refnum<vi>)
        n422 = control-ref of="Com_Mode_Trig Enable"() -> (w727:refnum<vi>)
        n423 = control-ref of="Com_Mode_Int Enable"() -> (w726:refnum<vi>)
        n424 = control-ref of="Com_ACT_CAL F0"() -> (w722:refnum<vi>)
        n425 = control-ref of="Com 2_FIFO_Size"() -> (w714:refnum<vi>)
        n426 = control-ref of="Com 2_FIFO_Full Level"() -> (w713:refnum<vi>)
        n427 = control-ref of="Com 2_FIFO_Empty Level"() -> (w712:refnum<vi>)
        n428 = control-ref of="Com_Mode_Play Mode"() -> (w728:refnum<vi>)
        n429 = control-ref of="Com_PWM_Mode"() -> (w725:refnum<vi>)
        n430 = control-ref of="Com_PWM_Freq"() -> (w724:refnum<vi>)
        n431 = control-ref of="Com_VD Clamp"() -> (w723:refnum<vi>)
        n432 = control-ref of="Com_ACT_F0 In"() -> (w721:refnum<vi>)
        n433 = control-ref of="Com_ACT_Freq Range"() -> (w720:refnum<vi>)
        n434 = control-ref of="Com 2_ZXD_Null Time"() -> (w718:refnum<vi>)
        n435 = control-ref of="Com 2_ZXD_GND Time"() -> (w717:refnum<vi>)
        n436 = control-ref of="Com 2_ZXD_BEMF Gain"() -> (w716:refnum<vi>)
        n437 = control-ref of="Com 2_ZXD_Sense Time"() -> (w715:refnum<vi>)
        n438 = Build Array(w728, w727, w726, w725, w724, w723, w722, w721, w720) -> (w689:refnum<vi>[])
        n439 = Build Array(w719, w718, w717, w716, w715, w714, w713, w712) -> (w688:refnum<vi>[])
        n440 = control-ref of="Mem_Wave Seq"() -> (w711:refnum<vi>)
        n441 = control-ref of="Mem/AT_Brake Ctrl"() -> (w707:refnum<vi>)
        n442 = control-ref of="Mem_Wave Seq Ctrl_Mute"() -> (w710:refnum<vi>)
        n443 = control-ref of="AT_Track_Pattern"() -> (w706:refnum<vi>)
        n444 = control-ref of="AT_Track_OD Enable"() -> (w701:refnum<vi>)
        n445 = control-ref of="Trig_Ctrl_Restart Enable"() -> (w698:refnum<vi>)
        n446 = control-ref of="Trig_Ctrl_Tirg Mode"() -> (w697:refnum<vi>)
        n447 = control-ref of="Trig_Ctrl_Trig Level"() -> (w696:refnum<vi>)
        n448 = control-ref of="Trig_Ctrl_Trig Priority"() -> (w695:refnum<vi>)
        n449 = control-ref of="Trig_Wave_R_Enable"() -> (w693:refnum<vi>)
        n450 = control-ref of="Trig_Wave_F_Enable"() -> (w692:refnum<vi>)
        n451 = control-ref of="Mem_Wave Seq Ctrl_Gain"() -> (w709:refnum<vi>)
        n452 = control-ref of="Mem_Wave Seq Ctrl_Loop"() -> (w708:refnum<vi>)
        n453 = control-ref of="AT_Track_Loop"() -> (w705:refnum<vi>)
        n454 = control-ref of="AT_Track_Play"() -> (w704:refnum<vi>)
        n455 = control-ref of="AT_Track_Idle"() -> (w703:refnum<vi>)
        n456 = control-ref of="AT_Track_Shape"() -> (w702:refnum<vi>)
        n457 = control-ref of="AT_Track_OD Level"() -> (w700:refnum<vi>)
        n458 = control-ref of="AT_Track_OD Cycle"() -> (w699:refnum<vi>)
        n459 = control-ref of="Trig_Ctrl_Interval"() -> (w694:refnum<vi>)
        n460 = control-ref of="Trig_Wave_R"() -> (w691:refnum<vi>)
        n461 = control-ref of="Trig_Wave_F"() -> (w690:refnum<vi>)
        n462 = property class="VI"() -> ("Panel"=w683:refnum<vi>)  [unwired: 2 in, 2 out]
        n463 = Build Array(w711, w710, w709, w708, w707) -> (w687:refnum<vi>[])
        n464 = Build Array(w706, w705, w704, w703, w702, w701, w700, w699) -> (w686:refnum<vi>[])
        n465 = Build Array(w698, w697, w696, w695, w694, w693, w692, w691, w690) -> (w685:refnum<vi>[])
        n466 = property class="Pnl"(reference=w683, "DeferPanUpdts"=TRUE ("패널 업데이트 연기")) -> (reference out=w679:refnum<vi>, error out=w681:errorcluster)  [unwired: 1 in]
        n467 = Build Array (concatenate)(w689, w688, w687, w686, w685) -> (w684:refnum<vi>[])
        n468 = for {
          tunnel: w684 -> [w744] mode=indexing
          shift-right: [w742] -> w680
          shift-left: w681 -> [w743]
          n469 = invoke class="Ctl" method="Reinit To Default"(reference=w744, error in=w743) -> (error out=w742:errorcluster)  [unwired: 1 in, 2 out]
        }
        n470 = property class="Pnl"(reference=w679, error in=w680, "DeferPanUpdts"=FALSE ("패널 업데이트 연기")) -> ()  [unwired: 2 out]
      }
      event Value Change {
        w750 = u32 18 ("숫자형 텍스트.크기:높이")
        w754 = refnum<vi> refnum  # 디지털
        w765 = refnum<vi> refnum  # 클러스터
        # "Hidden, Fuse 페이지에서 Data Size (8bit, 16bit) 선택에 따라\nRead, Write 숫자형 컨트롤의 16진수 자릿수와 최대값 설정"
        # "W Data"
        # "R Data"
        n471 = event-data() -> ("CtlRef"=w767:refnum<vi>, "NewVal"=w759:u16)  [unwired: 1 in, 4 out]
        n472 = To Unsigned Byte Integer(number=w759) -> (unsigned 8bit integer=w748:u8)
        n473 = property class="Ring (엄격한)"(reference=w767) -> ("Owner"=w752:refnum<vi>)  [unwired: 1 in, 2 out]
        n474 = Multiply(x=w748, y=u8 2) -> (x*y=w757:u8)
        n475 = Multiply(x=w748, y=u8 8) -> (x*y=w747:u8)
        n476 = Format Into String(format string="%%0%0dx" ("포맷 문자열"), w757) -> (resulting string=w753:string)  [unwired: 2 in, 1 out]
        n477 = Power Of 2(x=w747) -> (2^x=w746:dbl)
        n478 = To More Specific Class(target class=w765, reference=w752) -> (specific class reference=w766:refnum<vi>)  [unwired: 1 in, 1 out]
        n479 = Decrement(x=w746) -> (x-1=w745:dbl)
        n480 = property class="Clust"(reference=w766) -> ("Controls[]"=w764:refnum<vi>[])  [unwired: 1 in, 2 out]
        n481 = Index Array(array=w764, index #1=3 ("인덱스"), index #2=5 ("인덱스")) -> (element #1=w761:refnum<vi>, element #2=w751:refnum<vi>)
        n482 = To More Specific Class(target class=w754, reference=w761) -> (specific class reference=w760:refnum<vi>)  [unwired: 1 in, 1 out]
        n483 = To More Specific Class(target class=w754, reference=w751) -> (specific class reference=w755:refnum<vi>)  [unwired: 1 in, 1 out]
        n484 = property class="DigNum"(reference=w760, "FormatString"=w753, "NumText.Height"=w750) -> ()  [unwired: 1 in, 2 out]
        n485 = property class="DigNum"(reference=w755, "FormatString"=w753, "NumText.Height"=w750, "Maximum"=w745) -> ()  [unwired: 1 in, 2 out]
      }
      event Value Change {
        w779 = refnum<vi> refnum  # 디지털
        # "Hidden, Fuse 페이지에서 R 버튼 클릭 시 I2C Read 실행"
        n486 = event-data() -> ("CtlRef"=w785:refnum<vi>)  [unwired: 1 in, 5 out]
        n487 = property class="Bool"(reference=w785) -> ("Owner"=w778:refnum<vi>)  [unwired: 1 in, 2 out]
        n488 = control-ref of="Register 1"() -> (w777:refnum<vi>)
        n489 = To More Specific Class(target class=w777, reference=w778) -> (specific class reference=w784:refnum<vi>)  [unwired: 1 in, 1 out]
        n490 = property class="Clust"(reference=w784) -> ("Controls[]"=w783:refnum<vi>[], "Value"=w775:variant)  [unwired: 1 in, 2 out]
        n491 = Variant To Data(type=T10 {"Addr"=0, "Name"="", "Data Size"=0, "R Data"=0, "R Btn"=FALSE, "W Data"=0, "W Btn"=FALSE} ("클러스터"), Variant=w775) -> (data=w774:T10)  [unwired: 1 in, 1 out]
        n492 = Index Array(array=w783, index=3 ("인덱스")) -> (element=w781:refnum<vi>)
        n493 = Unbundle By Name(w774) -> ("Addr"=w771:u8, "Data Size"=w769:u16)
        n494 = To More Specific Class(target class=w779, reference=w781) -> (specific class reference=w780:refnum<vi>)  [unwired: 1 in, 1 out]
        n495 = global read "(Var)System Variables.vi" "Main VI Log Ref"() -> (w772:refnum<vi>)
        n496 = global read "(Var)System Variables.vi" "IC I2C ID"() -> (w773:u8)
        n497 = call-poly "(SubVI)I2C.vi"("Log Ref"=w772, "Size to Read"=w769, "Start Address"=w771, "ID"=w773) -> ("Read Data"=w770:u8[])  [unwired: 5 in, 2 out]
        n498 = case shown="2" w769 {
          tunnel: w770 -> [w787 w790]
          tunnel: [w786 w788] -> w768
          frame 1, Default {
            n499 = Index Array(array=w787) -> (element=w786:u8)  [unwired: 1 in]
          }
          frame 2 {
            n500 = Type Cast(type=u16 0 ("타입"), x=w790) -> (*(type *) &x=w788:u16)
          }
        }
        n501 = property class="DigNum"(reference=w780, "Value"=w768) -> ()  [unwired: 1 in, 2 out]
      }
      event Value Change {
        # "Hidden, Fuse 페이지에서 W 버튼 클릭 시 I2C Write 실행"
        n502 = event-data() -> ("CtlRef"=w803:refnum<vi>)  [unwired: 1 in, 5 out]
        n503 = property class="Bool"(reference=w803) -> ("Owner"=w801:refnum<vi>)  [unwired: 1 in, 2 out]
        n504 = control-ref of="Register 1"() -> (w800:refnum<vi>)
        n505 = To More Specific Class(target class=w800, reference=w801) -> (specific class reference=w802:refnum<vi>)  [unwired: 1 in, 1 out]
        n506 = property class="Clust"(reference=w802) -> ("Value"=w798:variant)  [unwired: 1 in, 2 out]
        n507 = Variant To Data(type=T10 {"Addr"=0, "Name"="", "Data Size"=0, "R Data"=0, "R Btn"=FALSE, "W Data"=0, "W Btn"=FALSE} ("클러스터"), Variant=w798) -> (data=w797:T10)  [unwired: 1 in, 1 out]
        n508 = Unbundle By Name(w797) -> ("Addr"=w794:u8, "Data Size"=w793:u16, "W Data"=w792:u16)
        n509 = case shown="2" w793 {
          tunnel: [w804 w808] -> w791
          tunnel: w792 -> [w806 w809]
          frame 1, Default {
            n510 = To Unsigned Byte Integer(number=w806) -> (unsigned 8bit integer=w805:u8)
            n511 = Build Array(w805) -> (w804:u8[])
          }
          frame 2 {
            n512 = Type Cast(type=u8[] [] ("타입"), x=w809) -> (*(type *) &x=w808:u8[])
          }
        }
        n513 = global read "(Var)System Variables.vi" "Main VI Log Ref"() -> (w795:refnum<vi>)
        n514 = global read "(Var)System Variables.vi" "IC I2C ID"() -> (w796:u8)
        n515 = call-poly "(SubVI)I2C.vi"("Log Ref"=w795, "Data to Write"=w791, "Start Address"=w794, "ID"=w796) -> ()  [unwired: 6 in, 2 out]
      }
      event Key Down? {
        # "Hidden, Fuse 탭의 Read 숫자형은\n클러스터 컨트롤 안에 있기 때문에 인디케이터로 설정 불가능\n컨트롤이지만 인디케이터처럼 동작하기 위해 키 입력을 버림\n\n키 입력을 버려도 Ctrl+C의 경우 사용 가능함"
        n516 = event-data() -> ()  [unwired: 1 in, 10 out]
        n517 = event-data("Discard?"=TRUE ("버림?")) -> ()  [unwired: 6 in, 1 out]
      }
      event "Script_Path": Value Change {
        # "Script 페이지에서 파일 경로가 비어있으면 Run 버튼 비활성화"
        n518 = event-data() -> ()  [unwired: 1 in, 6 out]
        n519 = property on="Script_Run Btn" class="Clust"() -> ("Controls[]"=w811:refnum<vi>[])  [unwired: 2 in, 2 out]
        n520 = Cluster To Array(cluster="Script_Path") -> (array=w813:path[])
        n521 = for {
          tunnel: w813 -> [w819] mode=indexing
          tunnel: w811 -> [w818] mode=indexing
          n522 = Empty String/Path?(string/path=w819) -> (empty?=w817:bool)
          n523 = Select(t=T15."Disabled and Grayed Out", s=w817, f=T15."Enabled" ("비활성화")) -> (s? t:f=w814:T15)
          n524 = property class="Ctl"(reference=w818, "DisabledEnum"=w814) -> ()  [unwired: 1 in, 2 out]
        }
      }
      event "Script_Run Btn": Value Change {
        w824 = refnum<vi> refnum  # 경로
        # "Run 버튼 클릭 시 스크립트 파일 실행\nI2C Master 2 참고"
        n525 = event-data() -> ()  [unwired: 1 in, 6 out]
        n526 = Cluster To Array(cluster="Script_Run Btn") -> (array=w822:bool[])
        n527 = call "Search Unsorted 1D Array.vim"("element"=TRUE, "unsorted 1D array"=w822) -> ("index of element"=w827:i32)  [unwired: 9 in]
        n528 = property on="Script_Path" class="Clust (엄격한)"() -> (error out=w826:errorcluster, "Controls[]"=w830:refnum<vi>[])  [unwired: 2 in, 1 out]
        n529 = Index Array(array=w830, index=w827) -> (element=w829:refnum<vi>)
        n530 = To More Specific Class(target class=w824, reference=w829, error in=w826) -> (specific class reference=w828:refnum<vi>, error out=w825:errorcluster)
        n531 = property class="Path"(reference=w828, error in=w825) -> ("Value"=w823:path)  [unwired: 2 out]
        n532 = call "(SubVI)Run Script.vi"("GUI Log Obj"=w820, "Script File"=w823) -> ()  [unwired: 9 in, 1 out]
      }
      event Value Change {
        # "Wave Seq. 0 주소\n원소의 인덱스에 따라 주소를 증가"
        n533 = event-data() -> ("CtlRef"=w844:refnum<vi>)  [unwired: 1 in, 5 out]
        n534 = property class="Clust (엄격한)"(reference=w844) -> (reference out=w833:refnum<vi>, "Value"=w832:T4)  [unwired: 1 in, 1 out]
        n535 = control-ref of="Mem Set_Wave Seq Loop"() -> (w834:refnum<vi>)
        n536 = Unbundle(w832) -> ("Mode"=w836:u8, "Seq/Delay"=w841:u8)
        n537 = call "(DW7912)Update Wave Seq Value Ring.vi"("Wave Seq Loop Ref In"=w834, "Wave Seq Ref In"=w833) -> ("index"=w835:u8)  [unwired: 8 in, 1 out]
        n538 = Logical Shift(y=i16 7, x=w836) -> (x << y=w842:u8)
        n539 = Or(x=w842, y=w841) -> (x .or. y?=w840:u8)
        n540 = Add(x=w835, y=u8 15) -> (x+y=w839:u8)
        n541 = global read "(Var)System Variables.vi" "Main VI Log Ref"() -> (w837:refnum<vi>)
        n542 = global read "(Var)System Variables.vi" "IC I2C ID"() -> (w838:u8)
        n543 = call-poly "(SubVI)I2C.vi"("Log Ref"=w837, "Data to Write"=w840, "Address"=w839, "ID"=w838) -> ()  [unwired: 6 in, 2 out]
      }
      event Value Change {
        w851 = refnum<vi> refnum  # 클러스터
        # "FAE3팀에서 Wave Seq.의 Mode 변경 시 \nMem.No의 값을 0으로 변경하도록 요청"
        n544 = event-data() -> ("CtlRef"=w846:refnum<vi>)  [unwired: 1 in, 5 out]
        n545 = property class="Ring (엄격한)"(reference=w846) -> ("Owner"=w853:refnum<vi>)  [unwired: 1 in, 2 out]
        n546 = To More Specific Class(target class=w851, reference=w853) -> (specific class reference=w852:refnum<vi>)  [unwired: 1 in, 1 out]
        n547 = property class="Clust"(reference=w852) -> ("Controls[]"=w850:refnum<vi>[])  [unwired: 1 in, 2 out]
        n548 = Index Array(array=w850, index=1 ("인덱스")) -> (element=w848:refnum<vi>)
        n549 = property class="Ctl"(reference=w848, "Value"=u8 0) -> ()  [unwired: 1 in, 2 out]
      }
      event "Mem Set_Wave Seq Loop.Loop 0", "Mem Set_Wave Seq Loop.Loop 1", "Mem Set_Wave Seq Loop.Loop 2", "Mem Set_Wave Seq Loop.Loop 3", "Mem Set_Wave Seq Loop.Loop 4", "Mem Set_Wave Seq Loop.Loop 5", "Mem Set_Wave Seq Loop.Loop 6", "Mem Set_Wave Seq Loop.Loop 7": Value Change {
        # "Wave Seq Loop의 경우 2개가 1바이트"
        n550 = event-data() -> ("CtlRef"=w865:refnum<vi>)  [unwired: 1 in, 5 out]
        n551 = property on="Mem Set_Wave Seq Loop" class="Clust (엄격한)"() -> ("Controls[]"=w870:refnum<vi>[])  [unwired: 2 in, 2 out]
        n552 = call "Search Unsorted 1D Array.vim"("element"=w865, "unsorted 1D array"=w870) -> ("index of element"=w869:i32)  [unwired: 9 in]
        n553 = Cluster To Array(cluster="Mem Set_Wave Seq Loop") -> (array=w862:u8[])
        n554 = To Unsigned Byte Integer(number=w869) -> (unsigned 8bit integer=w871:u8)
        n555 = Quotient & Remainder(x=w871, y=u8 2) -> (floor(x/y)=w861:u8)  [unwired: 1 out]
        n556 = Multiply(x=w861, y=u8 2) -> (x*y=w855:u8)
        n557 = Add(x=w861, y=u8 23) -> (x+y=w868:u8)
        n558 = Index Array(array=w862, index #1=w855) -> (element #1=w858:u8, element #2=w860:u8)  [unwired: 1 in]
        n559 = global read "(Var)System Variables.vi" "Main VI Log Ref"() -> (w866:refnum<vi>)
        n560 = global read "(Var)System Variables.vi" "IC I2C ID"() -> (w867:u8)
        n561 = Logical Shift(y=i16 4, x=w860) -> (x << y=w857:u8)
        n562 = Or(x=w858, y=w857) -> (x .or. y?=w856:u8)
        n563 = call-poly "(SubVI)I2C.vi"("Log Ref"=w866, "Data to Write"=w856, "Address"=w868, "ID"=w867) -> ()  [unwired: 6 in, 2 out]
      }
      event "Mem_Main Seq Loop": Value Change {
        n564 = event-data() -> ()  [unwired: 1 in, 6 out]
        n565 = global read "(Var)System Variables.vi" "Main VI Log Ref"() -> (w875:refnum<vi>)
        n566 = global read "(Var)System Variables.vi" "IC I2C ID"() -> (w876:u8)
        n567 = call-poly "(SubVI)I2C.vi"("Log Ref"=w875, "Data to Write"="Mem_Main Seq Loop", "Address"=u8 27, "ID"=w876) -> ()  [unwired: 6 in, 2 out]
      }
      event "Mem_Start", "Mem_Stop", "AT_Start", "AT_Stop": Value Change {
        # "Stop 이벤트 시 0\nStart 이벤트 시 1"
        n568 = event-data() -> ()  [unwired: 1 in, 6 out]
        n569 = Or(x="Mem_Start", y="AT_Start") -> (x .or. y?=w878:bool)
        n570 = Boolean To (0,1)(Boolean=w878) -> (0, 1=w881:i16)
        n571 = To Unsigned Byte Integer(number=w881) -> (unsigned 8bit integer=w880:u8)
        n572 = global read "(Var)System Variables.vi" "Main VI Log Ref"() -> (w883:refnum<vi>)
        n573 = global read "(Var)System Variables.vi" "IC I2C ID"() -> (w884:u8)
        n574 = call-poly "(SubVI)I2C.vi"("Log Ref"=w883, "Data to Write"=w880, "Address"=u8 12, "ID"=w884) -> ()  [unwired: 6 in, 2 out]
      }
      event "MEM/AT_AB.Shape", "MEM/AT_AB.OD Enable", "MEM/AT_AB.OD Level", "MEM/AT_AB.OD Cycle", "MEM/AT_AB.Enable": Value Change {
        n575 = local read "MEM/AT_AB"() -> (w894:T1)
        n576 = event-data() -> ()  [unwired: 1 in, 6 out]
        n577 = Unbundle By Name(w894) -> ("OD Cycle"=w893:u8, "OD Level"=w892:u8, "OD Enable"=w891:bool, "Shape"=w890:u8, "Enable"=w887:bool)
        n578 = Boolean To (0,1)(Boolean=w891) -> (0, 1=w905:i16)
        n579 = Boolean To (0,1)(Boolean=w887) -> (0, 1=w888:i16)
        n580 = To Unsigned Byte Integer(number=w905) -> (unsigned 8bit integer=w902:u8)
        n581 = To Unsigned Byte Integer(number=w888) -> (unsigned 8bit integer=w886:u8)
        n582 = Logical Shift(y=i16 0, x=w893) -> (x << y=w900:u8)
        n583 = Logical Shift(y=i16 2, x=w892) -> (x << y=w897:u8)
        n584 = Logical Shift(y=i16 4, x=w902) -> (x << y=w896:u8)
        n585 = Logical Shift(y=i16 5, x=w890) -> (x << y=w895:u8)
        n586 = Logical Shift(y=i16 7, x=w886) -> (x << y=w885:u8)
        n587 = global read "(Var)System Variables.vi" "Main VI Log Ref"() -> (w907:refnum<vi>)
        n588 = global read "(Var)System Variables.vi" "IC I2C ID"() -> (w908:u8)
        n589 = Compound Arithmetic op=OR(w900, w897, w896, w895, w885) -> (w901:u8)
        n590 = call-poly "(SubVI)I2C.vi"("Log Ref"=w907, "Data to Write"=w901, "Address"=u8 7, "ID"=w908) -> ()  [unwired: 6 in, 2 out]
      }
      event "MEM/AT_AB.Gain": Value Change {
        n591 = event-data() -> ("NewVal"=w909:u8)  [unwired: 1 in, 5 out]
        n592 = global read "(Var)System Variables.vi" "Main VI Log Ref"() -> (w911:refnum<vi>)
        n593 = global read "(Var)System Variables.vi" "IC I2C ID"() -> (w912:u8)
        n594 = call-poly "(SubVI)I2C.vi"("Log Ref"=w911, "Data to Write"=w909, "Address"=u8 8, "ID"=w912) -> ()  [unwired: 6 in, 2 out]
      }
      event "AT_Track_Pattern", "AT_Track_Loop": Value Change {
        n595 = event-data() -> ()  [unwired: 1 in, 6 out]
        n596 = Boolean To (0,1)(Boolean="AT_Track_Pattern") -> (0, 1=w921:i16)
        n597 = To Unsigned Byte Integer(number=w921) -> (unsigned 8bit integer=w916:u8)
        n598 = Logical Shift(y=i16 0, x="AT_Track_Loop") -> (x << y=w914:u8)
        n599 = Logical Shift(y=i16 7, x=w916) -> (x << y=w913:u8)
        n600 = global read "(Var)System Variables.vi" "Main VI Log Ref"() -> (w923:refnum<vi>)
        n601 = global read "(Var)System Variables.vi" "IC I2C ID"() -> (w924:u8)
        n602 = Compound Arithmetic op=OR(w914, w913) -> (w915:u8)
        n603 = call-poly "(SubVI)I2C.vi"("Log Ref"=w923, "Data to Write"=w915, "Address"=u8 30, "ID"=w924) -> ()  [unwired: 6 in, 2 out]
      }
      event "AT_Track_Play", "AT_Track_Idle": Value Change {
        n604 = event-data() -> ("CtlRef"=w927:refnum<vi>, "NewVal"=w925:u8)  [unwired: 1 in, 4 out]
        n605 = property class="Ring (엄격한)"(reference=w927) -> ("Label.Text"=w928:string)  [unwired: 1 in, 2 out]
        n606 = case shown="\"AT_Track_Play\", 기본" w928 {
          tunnel: [u8 31 u8 32] -> w926
          frame "AT_Track_Play", Default {
          }
          frame "AT_Track_Idle" {
          }
        }
        n607 = global read "(Var)System Variables.vi" "Main VI Log Ref"() -> (w929:refnum<vi>)
        n608 = global read "(Var)System Variables.vi" "IC I2C ID"() -> (w930:u8)
        n609 = call-poly "(SubVI)I2C.vi"("Log Ref"=w929, "Data to Write"=w925, "Address"=w926, "ID"=w930) -> ()  [unwired: 6 in, 2 out]
      }
      event "AT_Track_Shape", "AT_Track_OD Enable", "AT_Track_OD Level", "AT_Track_OD Cycle": Value Change {
        n610 = event-data() -> ()  [unwired: 1 in, 6 out]
        n611 = Boolean To (0,1)(Boolean="AT_Track_OD Enable") -> (0, 1=w947:i16)
        n612 = To Unsigned Byte Integer(number=w947) -> (unsigned 8bit integer=w944:u8)
        n613 = Logical Shift(y=i16 0, x="AT_Track_OD Cycle") -> (x << y=w942:u8)
        n614 = Logical Shift(y=i16 2, x="AT_Track_OD Level") -> (x << y=w935:u8)
        n615 = Logical Shift(y=i16 4, x=w944) -> (x << y=w934:u8)
        n616 = Logical Shift(y=i16 5, x="AT_Track_Shape") -> (x << y=w933:u8)
        n617 = global read "(Var)System Variables.vi" "Main VI Log Ref"() -> (w949:refnum<vi>)
        n618 = global read "(Var)System Variables.vi" "IC I2C ID"() -> (w950:u8)
        n619 = Compound Arithmetic op=OR(w942, w935, w934, w933) -> (w943:u8)
        n620 = call-poly "(SubVI)I2C.vi"("Log Ref"=w949, "Data to Write"=w943, "Address"=u8 6, "ID"=w950) -> ()  [unwired: 6 in, 2 out]
      }
      event "Com_ACT_CAL F0": Value Change {
        n621 = event-data() -> ()  [unwired: 1 in, 6 out]
        n622 = Boolean To (0,1)(Boolean="Com_ACT_CAL F0") -> (0, 1=w953:i16)
        n623 = To Unsigned Byte Integer(number=w953) -> (unsigned 8bit integer=w951:u8)
        n624 = global read "(Var)System Variables.vi" "Main VI Log Ref"() -> (w955:refnum<vi>)
        n625 = global read "(Var)System Variables.vi" "IC I2C ID"() -> (w956:u8)
        n626 = call-poly "(SubVI)I2C.vi"("Log Ref"=w955, "Data to Write"=w951, "Address"=u8 35, "ID"=w956) -> ()  [unwired: 6 in, 2 out]
      }
      event "Com_ACT_F0 In", "Com_ACT_Freq Range": Value Change {
        # "#7802_FPGA\nIC : 0x24\nFPGA : 0x3F"
        n627 = event-data() -> ()  [unwired: 1 in, 6 out]
        n628 = Logical Shift(y=i16 12, x="Com_ACT_Freq Range") -> (x << y=w961:u16)
        n629 = global read "(Var)System Variables.vi" "Main VI Log Ref"() -> (w965:refnum<vi>)
        n630 = global read "(Var)System Variables.vi" "IC I2C ID"() -> (w966:u8)
        n631 = Compound Arithmetic op=OR(w961, "Com_ACT_F0 In") -> (w958:u16)
        n632 = Type Cast(type=u8[] [] ("타입"), x=w958) -> (*(type *) &x=w957:u8[])
        n633 = call-poly "(SubVI)I2C.vi"("Log Ref"=w965, "Data to Write"=w957, "Start Address"=u8 36 ("Address"), "ID"=w966) -> ()  [unwired: 6 in, 2 out]
      }
      event "Trig_Ctrl_Trig Priority", "Trig_Ctrl_Interval", "Trig_Ctrl_Trig Level", "Trig_Ctrl_Tirg Mode", "Trig_Ctrl_Restart Enable": Value Change {
        n634 = event-data() -> ()  [unwired: 1 in, 6 out]
        n635 = Number To Boolean Array(number="Trig_Ctrl_Interval") -> (Boolean array=w977:bool[])
        n636 = Index Array(array=w977) -> (element #1=w975:bool, element #2=w974:bool, element #3=w973:bool)  [unwired: 3 in]
        n637 = global read "(Var)System Variables.vi" "Main VI Log Ref"() -> (w980:refnum<vi>)
        n638 = Build Array("Trig_Ctrl_Trig Priority", w975, w974, w973, "Trig_Ctrl_Trig Level", "Trig_Ctrl_Tirg Mode", FALSE, "Trig_Ctrl_Restart Enable") -> (w970:bool[])
        n639 = global read "(Var)System Variables.vi" "IC I2C ID"() -> (w981:u8)
        n640 = Boolean Array To Number ("불리언 배열을 숫자로")(Boolean array=w970) -> (number=w969:u8)
        n641 = call-poly "(SubVI)I2C.vi"("Log Ref"=w980, "Data to Write"=w969, "Address"=u8 4, "ID"=w981) -> ()  [unwired: 6 in, 2 out]
      }
      event "Trig_Wave_R_Enable", "Trig_Wave_R", "Trig_Wave_F_Enable", "Trig_Wave_F": Value Change {
        n642 = event-data() -> ("CtlRef"=w995:refnum<vi>)  [unwired: 1 in, 5 out]
        n643 = property class="Ctl"(reference=w995) -> ("Label.Text"=w996:string)  [unwired: 1 in, 2 out]
        n644 = case shown="\"Trig_Wave_R\", \"Trig_Wave_R_Enable\", 기본" w996 {
          tunnel: [u8 28 u8 29] -> w994
          tunnel: "Trig_Wave_R_Enable" -> [w1000 _]
          tunnel: "Trig_Wave_R" -> [w999 _]
          tunnel: "Trig_Wave_F_Enable" -> [_ w1003]
          tunnel: "Trig_Wave_F" -> [_ w1002]
          tunnel: [w1000 w1003] -> w989
          tunnel: [w999 w1002] -> w985
          frame "Trig_Wave_R", "Trig_Wave_R_Enable", Default {
          }
          frame "Trig_Wave_F", "Trig_Wave_F_Enable" {
          }
        }
        n645 = Not(x=w989) -> (.not. x?=w982:bool)
        n646 = Boolean To (0,1)(Boolean=w982) -> (0, 1=w988:i16)
        n647 = global read "(Var)System Variables.vi" "Main VI Log Ref"() -> (w997:refnum<vi>)
        n648 = To Unsigned Byte Integer(number=w988) -> (unsigned 8bit integer=w984:u8)
        n649 = global read "(Var)System Variables.vi" "IC I2C ID"() -> (w998:u8)
        n650 = Logical Shift(y=i16 7, x=w984) -> (x << y=w986:u8)
        n651 = Or(x=w986, y=w985) -> (x .or. y?=w983:u8)
        n652 = call-poly "(SubVI)I2C.vi"("Log Ref"=w997, "Data to Write"=w983, "Address"=w994, "ID"=w998) -> ()  [unwired: 6 in, 2 out]
      }
      event Value Change {
        # "Trigger 설정에 따른 그림 생성"
        # "비활성화, 시간 설정 범위 관련 처리"
        n653 = event-data() -> ("CtlRef"=w1009:refnum<vi>)  [unwired: 1 in, 5 out]
        n654 = call "(SubVI)Update Trigger Control Cluster.vi"("Trig Ctrl Ref"=w1009) -> ("Disable"=w1008:T15)  [unwired: 9 in, 1 out]
        n655 = property on="Trig_Gen_Set" class="Bool"("DisabledEnum"=w1008) -> ()  [unwired: 2 in, 2 out]
        n656 = call "(SubVI)GPIO Trigger Picture.vi"("num of ch (4)"=1, "Trig Ctrl"="Trig_Gen_Setting") -> ("picture"=→"Trig_Gen_Pict":picture)  [unwired: 9 in]
      }
      event "Trig_Gen_Set": Value Change {
        # "트리거 발생"
        n657 = event-data() -> ()  [unwired: 1 in, 6 out]
        n658 = local read "Trig_Gen_Setting"() -> (w1010:T6)
        n659 = call "(SubVI)System Command_Trig GPIO Control.vi"("Trig_Ctrl"=w1010) -> ()  [unwired: 10 in, 1 out]
      }
    }
    n660 = global read "(Var)System Variables.vi" "Quit System"() -> (w67:bool)
    n661 = Or(x="Stop", y=w67) -> (x .or. y?=w65:bool)
  }
  n662 = call-dynamic "release queue.vi"("GUI Log Class 입력"=w6) -> ()  [unwired: 9 in, 2 out]
  n663 = flat-sequence {
    tunnel: w44 -> [_]
    frame #0 {
      # "마지막 사용 값 저장"
      n664 = control-ref of="Trig_Gen_Setting"() -> (w1017:refnum<vi>)
      n665 = control-ref of="Hidden_Register Access"() -> (w1013:refnum<vi>)
      n666 = control-ref of="Fuse_Register Access"() -> (w1012:refnum<vi>)
      n667 = control-ref of="Script_Path"() -> (w1011:refnum<vi>)
      n668 = Build Array(w1017, w1013, w1012, w1011) -> (w1016:refnum<vi>[])
      n669 = call "(SubVI)Control Data_Save or Load Control Value.vi"("Common? (f)"=TRUE, "Function"=(Ctrl)Control_Data_Save_or_Load_Control_Data_Function."Save", "Control Ref"=w1016) -> ()  [unwired: 8 in, 1 out]
    }
  }
